vi "CIPT_softwarecontrol auto probe movement 9 8 23 - Copy.vi"() -> ()   [LabVIEW 2022 SP3]
uses:
  Git/CIPT/CIPT/Labview Project/CIPT modes.ctl
  <vilib>/Analysis/baseanly.llb/Mean (DBL).vi
  <vilib>/Utility/file.llb/Read Delimited Spreadsheet (DBL).vi
  <vilib>/Utility/file.llb/Read Delimited Spreadsheet (I64).vi
  <vilib>/gmath/NumericalOptimization/Nonlinear Curve Fit LM.vi
  <vilib>/Utility/file.llb/Write Delimited Spreadsheet (string).vi
  <vilib>/Utility/file.llb/Write Delimited Spreadsheet (I64).vi
  <vilib>/Utility/file.llb/Write Delimited Spreadsheet (DBL).vi
  C:/CIPT/Labview Project/Camera Driver/Labview Driver/OtherDrivers/LabVIEW/ueye.NET/uEyeDotNet.dll
  CIPT/Labview Project/Camera Driver/Labview Driver/OtherDrivers/LabVIEW/ueye.NET/uEyeDotNet.dll
  <vilib>/gmath/NI_Gmath.lvlib
  <instrlib>/Keithley DMM6500 DAQ6500 Series/Keithley DMM6500 DAQ6500 Series.lvlib
  <instrlib>/Keithley 24XX/Keithley 24XX.lvlib
  <instrlib>/Keithley 2182/Keithley 2182.lvlib
  <vilib>/Analysis/NI_AALBase.lvlib
panel:
  out "Resistance":sgl[](array[numeric])
  out "Comms Errors":errorcluster[](array[cluster])
  in  "Save File":bool
  out "error file out":errorcluster
  in  "output file path":path=path "C:/CIPT/Labview Project/csv files/test output.csv"
  in  "stop":bool
  in  "Tab Control":T1(tab)
  in  "Camera ID 3":enum16{"2", "1"}(ring)
  in  "Camera ID 1":enum16{"2", "1"}(ring)
  in  "down a2":bool
  in  "up a2":bool
  in  "down a1":bool
  in  "up a1":bool
  in  "down a3":bool
  in  "up a3":bool
  in  "down all":bool
  in  "up all":bool
  in  "steps /\n continuous \ntoggle":bool
  out "Image first camera":picture
  out "Serial Number 1":string
  in  "Init Camera":bool
  in  "Exit Camera":bool
  in  "Init Camera 2":bool
  in  "Exit Camera 2":bool
  out "Serial Number 2":string
  out "Image second camera":picture
  out "Error Camera 1":errorcluster caption="error"
  out "Error Camera 2":errorcluster caption="error"
  in  "COM 1":refnum<visa-resource-name>="COM1"
  out "error":errorcluster
  in  "Turn On Landing Test":bool
  in  "Step size":i32=10
  in  "Probe Landing File":path=path "C:/CIPT/Labview Project/csv files/Probe Landing cipt.csv"
  out "Probe List":i64[][](array[numeric])
  out "Resistance For Each Relay Setup":sgl[](array[numeric])
  in  "Probe Threshold (ohm)":dbl=100000.0
  out "Touching Probes":i64[][](array[numeric])
  in  "Auto Move Probe To Surface":bool
  out "Loaded":bool
  out "Loaded":bool
  out "Error Probe Configuration File":errorcluster
  in  "Probe Configuration File":path=path "C:/CIPT/Labview Project/csv files/test probe config.csv"
  in  "Probe Settings File":path=path "C:/CIPT/Labview Project/csv files/deafult_probe_setrings.CSV"
  out "Error Probe Settings File":errorcluster
  out "Probe Spacings":dbl[][](array[numeric])
  in  "Load":bool
  in  "Multiplexer":refnum<visa-resource-name>
  out "all rows":i64[][](array[numeric])
  out "Results Description":string[](array[string])
  out "Results":dbl[][](array[numeric])
  out "Probe Set 2":i32
  in  "Compliance voltage (V)":dbl=42.0
  in  "Measure Instrument":refnum<visa-resource-name>
  in  "Radio Buttons":T2 caption="Select Instrumentation"
  in  "Source Instrument":refnum<visa-resource-name>="Sourcemeter"
  in  "Run":bool
  in  "Current (µA)":dbl=10.0
  out "Measurement Log":string
  out "Probe Set":i32
  in  "Measurement Repeats":i32=10
  in  "Size Of Buffer Used For One Measurement":i32=3
  in  "Top Film R est.":dbl=0.25
  in  "Bottm Film R est.":dbl=0.25
  in  "RA est.":dbl=0.25
  out "Top Film R":dbl
  out "Bottom Film R":dbl
  out "RA":dbl
  out "error out (fitting model)":errorcluster
  in  "Fit Data":bool
  out "Measurements Map Out":map{string, dbl[]}(c390)
  # "Probe Landing cipt_probe check: checks probes individually \nProbe Landing cipt: checks for any connection"
  # "All"
  # "End"
  # "home"
  # "Delete"
  # "Insert"
  # "Page Down"
  # "Page up"
  # "F2"
  # "F1"
  # "Steps"
  # "Continuous"
  # "Probe Settings"
  # "Probe Configuration"
  # "I+"
  # "V+"
  # "V-"
  # "I-"
  # "Max Resolution of 2400 is 300 µV in 200 mV range"
  # "/"
  # "Sheet Resistance (RA)"
  # "Estimated Values"
  # "Fitted Values"
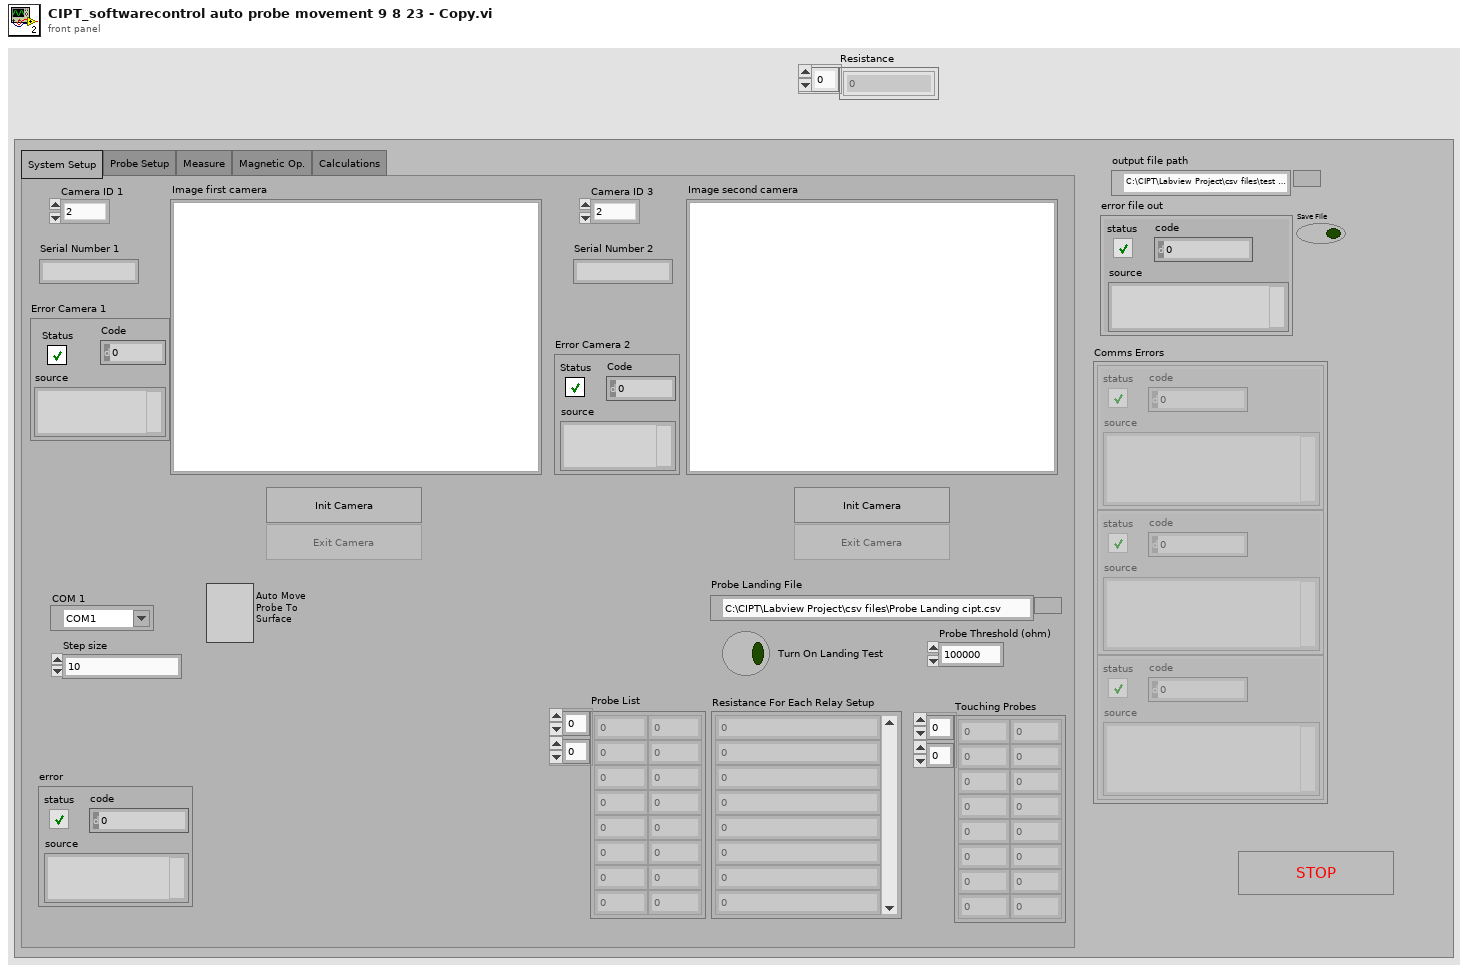
[diagram p1: front panel]
types:
  T1 = enum32{"System Setup", "Probe Setup", "Measure", "Magnetic Op.", "Calculations"}
  T2 = typedef "CIPT modes.ctl" = enum32{"DAQ6510", "2400 Only", "2400 and  2182", "SR830", "SR830 and 6221"}
  T3 = enum32{"System Setup", "Probe Setup", "Measure", "Magnetic Operations", "Calculations + Analyis"}
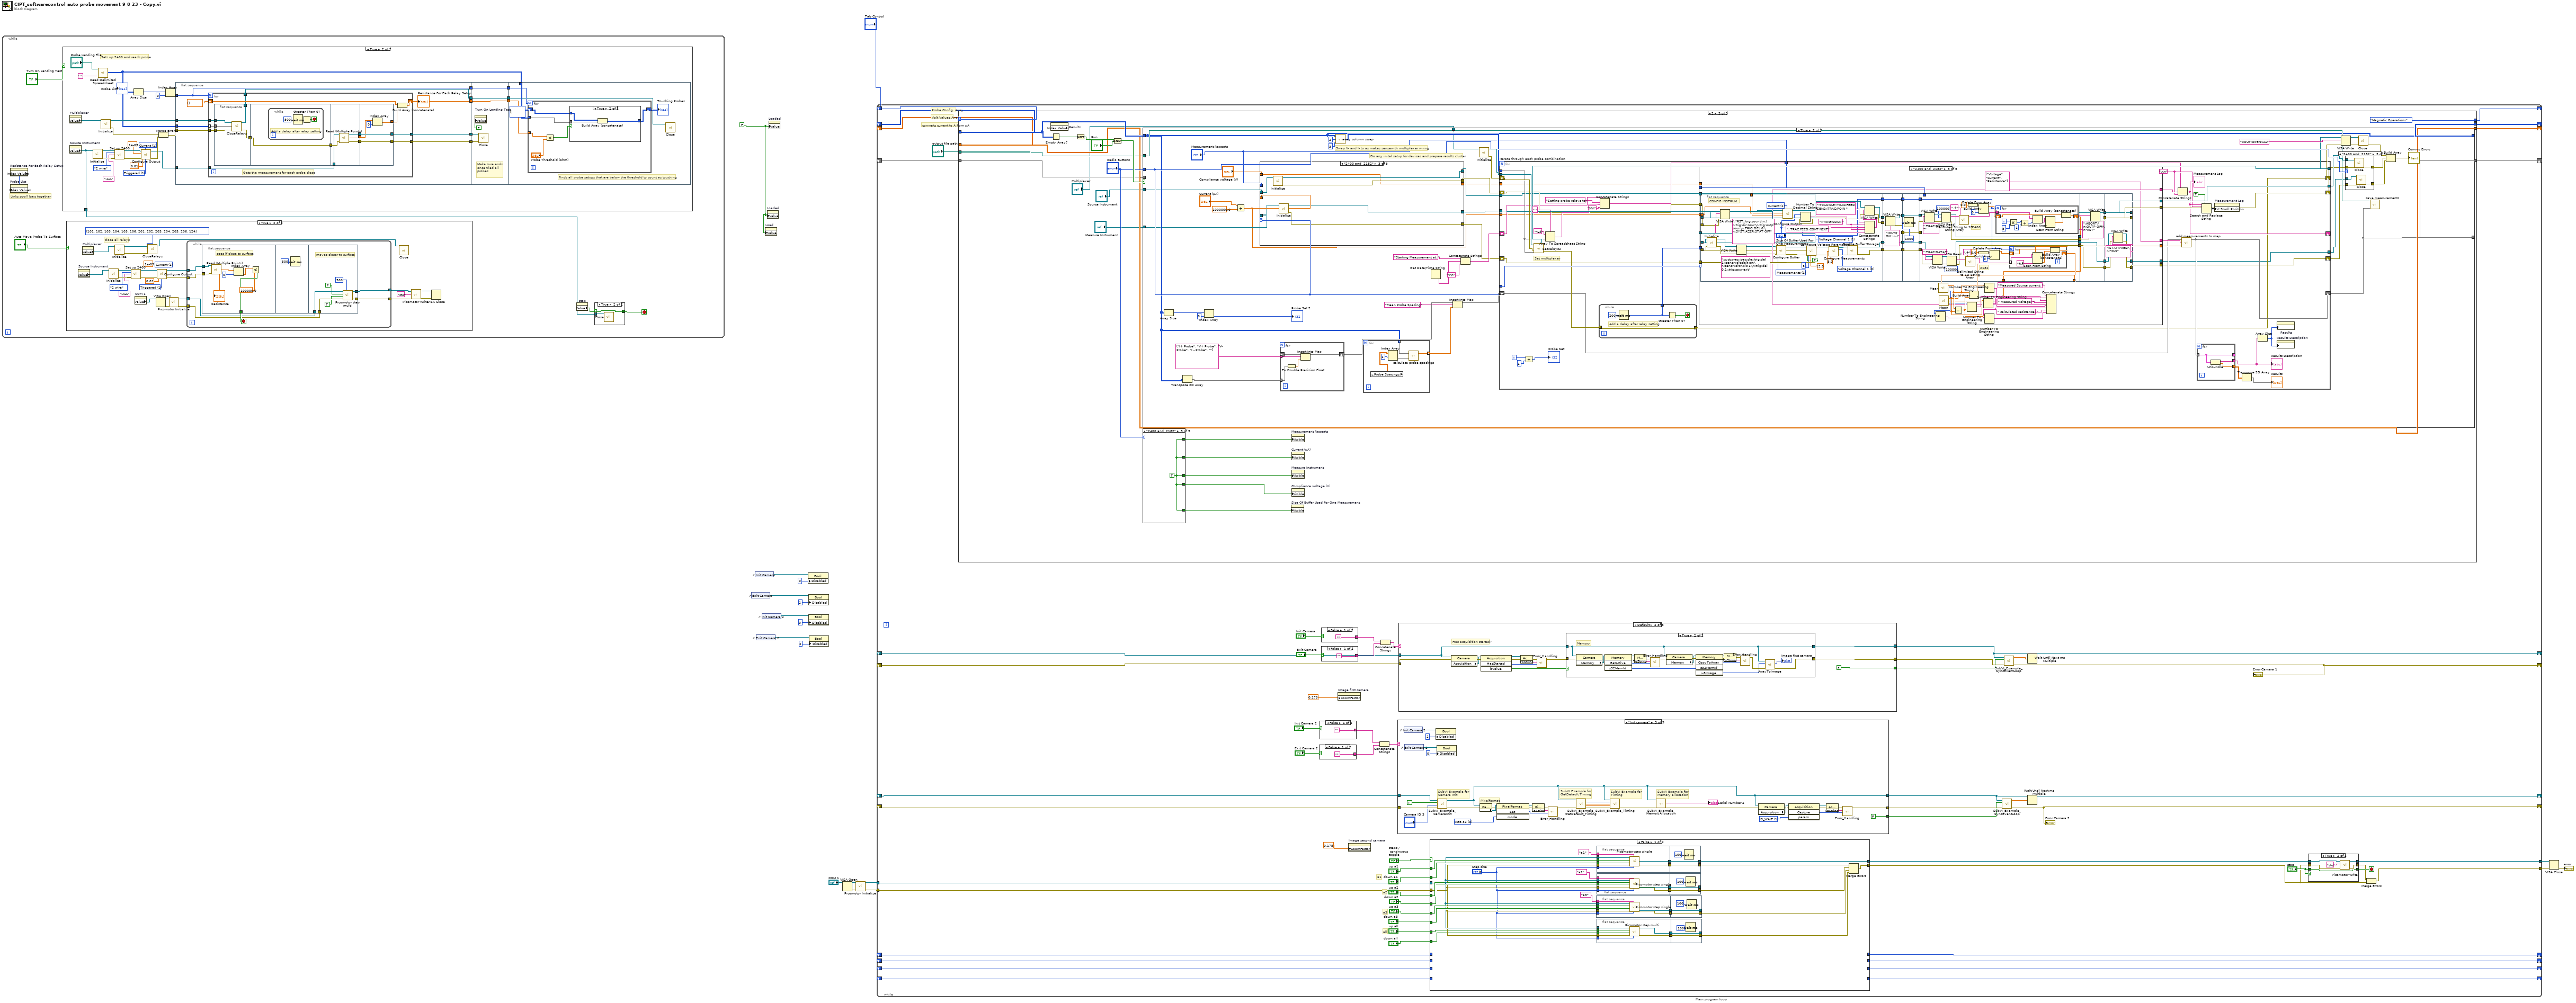
[diagram p0: block diagram]
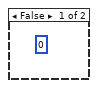
[diagram p4: hidden frame]
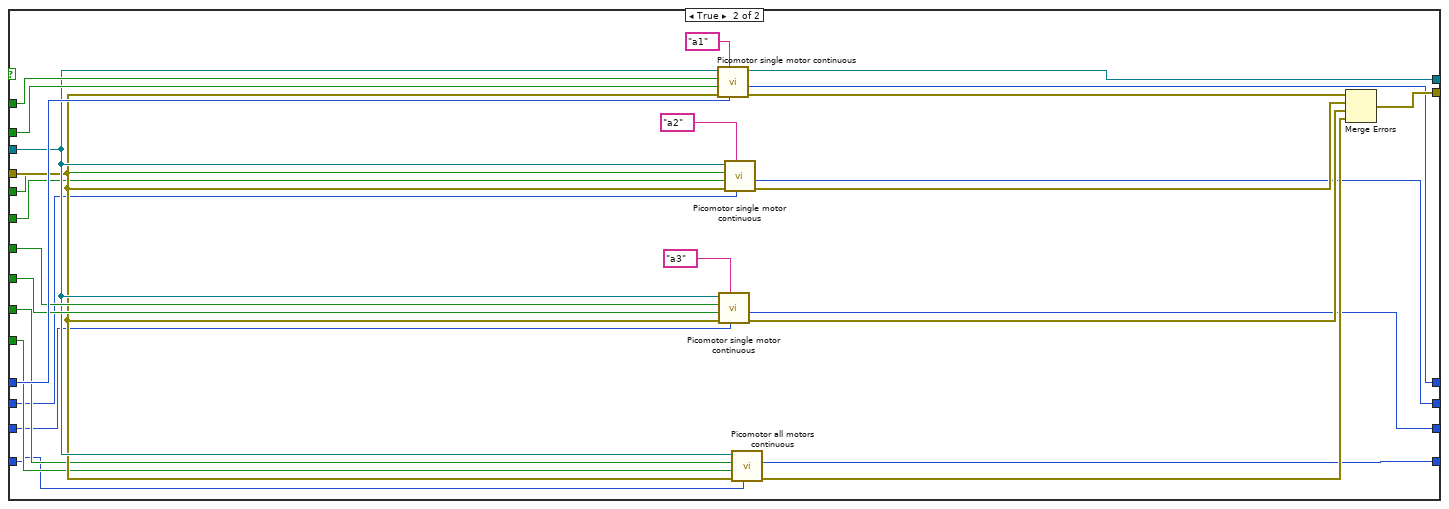
[diagram p6: hidden frame]
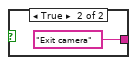
[diagram p8: hidden frame]
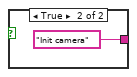
[diagram p9: hidden frame]
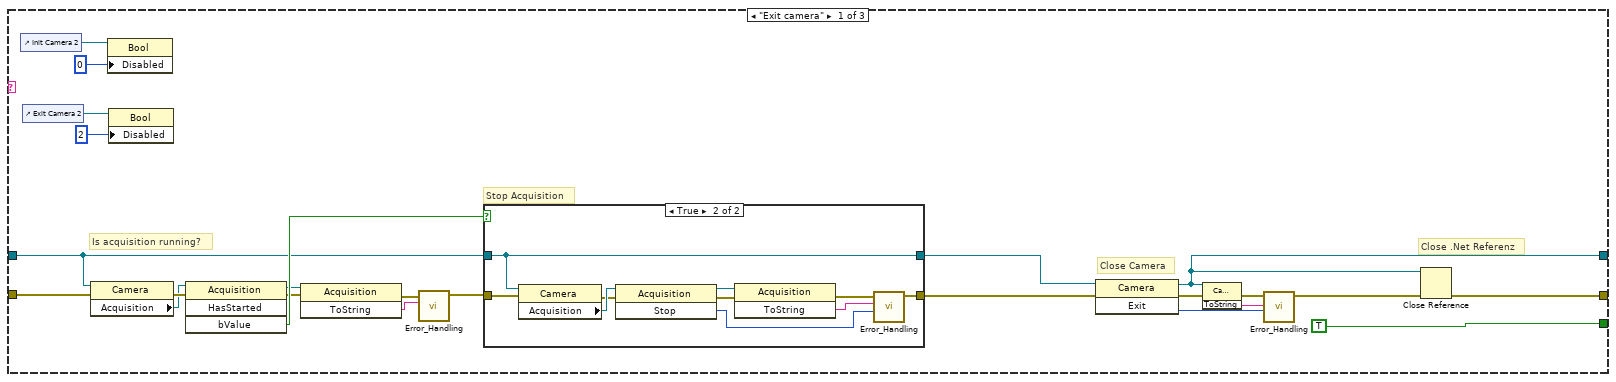
[diagram p10: hidden frame]
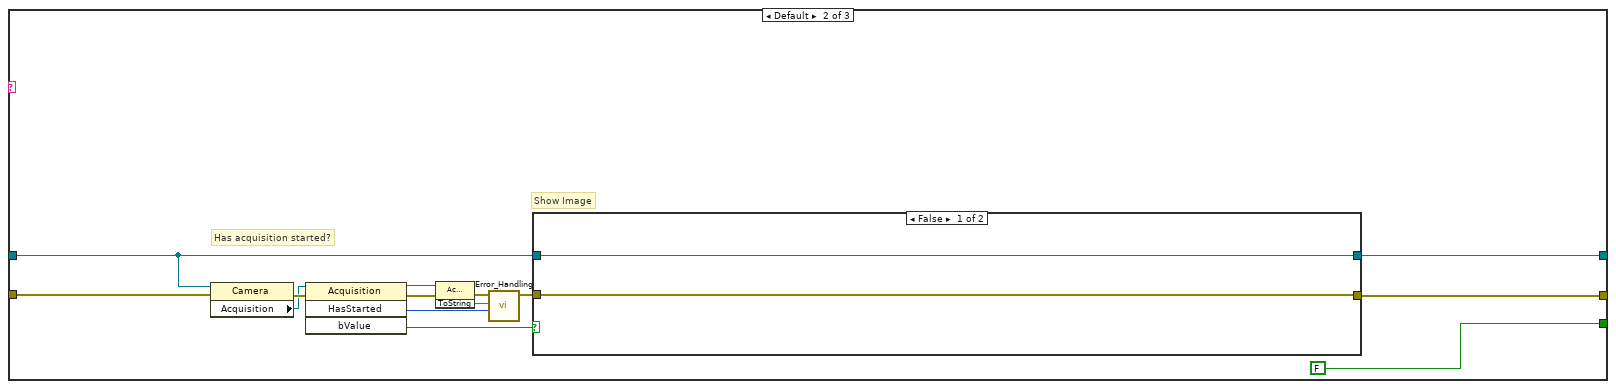
[diagram p12: hidden frame]
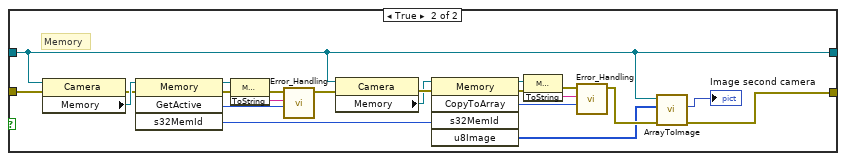
[diagram p13: hidden frame]
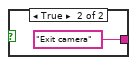
[diagram p14: hidden frame]
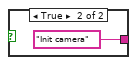
[diagram p15: hidden frame]
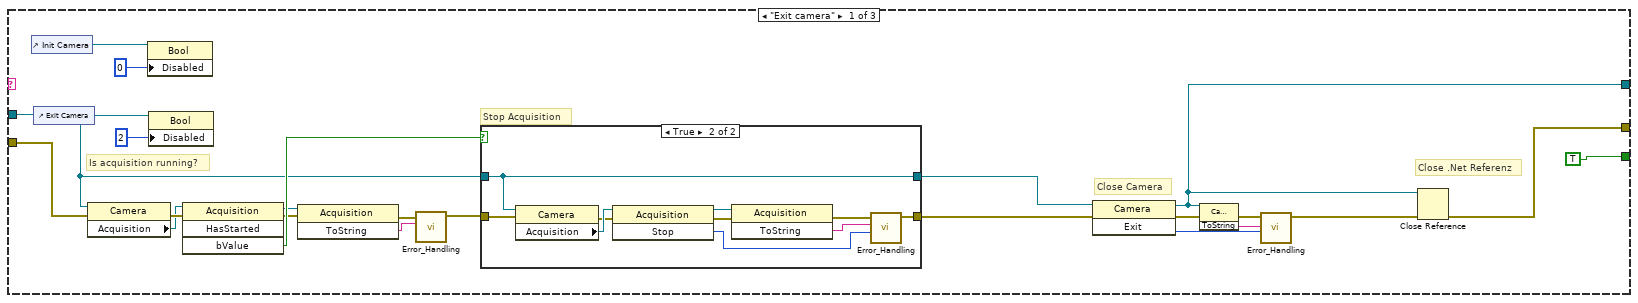
[diagram p16: hidden frame]
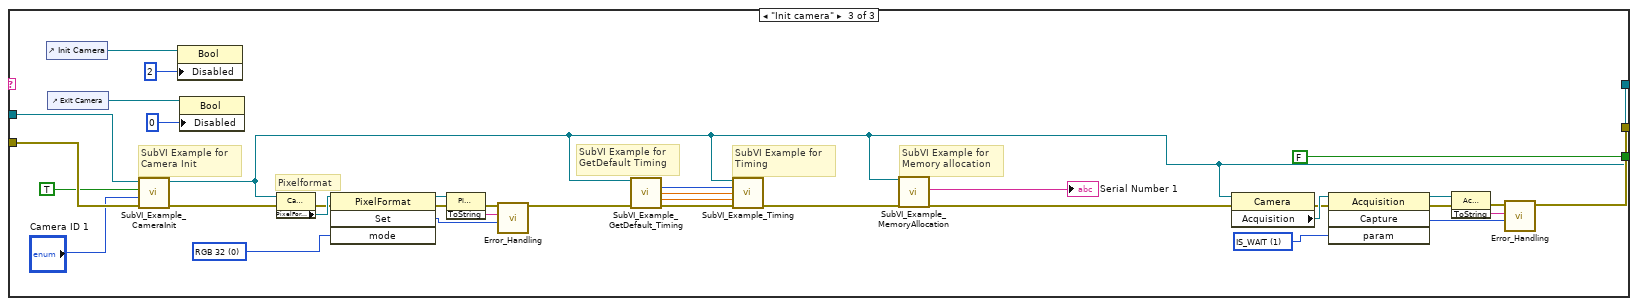
[diagram p19: hidden frame]
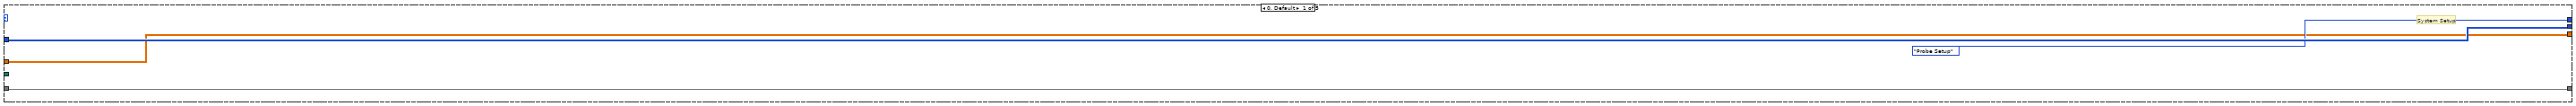
[diagram p20: hidden frame]
diagram:
  w9 = FALSE
  n1 = while {
    stop <- w24 stop-if-true
    # "Links scroll bars together"
    n2 = property on="Resistance For Each Relay Setup" class="Arr (strict)"() -> ("Index Values"=w20:u32[])  [unwired: 2 in, 2 out]
    n3 = property on="Probe List" class="Arr (strict)"("Index Values"=w20) -> ()  [unwired: 2 in, 2 out]
    n4 = case shown="True" "Turn On Landing Test" {
      tunnel: [_ w83] -> w21
      frame False {
        (unwired) 0
      }
      frame True {
        w100 = u16 1 items=["Immediate", "Triggered"] ("Output Type  (0: Immediate)")
        w99 = u16 1 items=["Voltage", "Current"] ("Source Mode  (0: Voltage)")
        # "Sets up 2400 and reads probe"
        n5 = property on="Multiplexer" class="VISAName"() -> ("Value"=w94:refnum<visa-resource-name>)  [unwired: 2 in, 2 out]
        n6 = property on="Source Instrument" class="VISAName"() -> ("Value"=w83:refnum<visa-resource-name>)  [unwired: 2 in, 2 out]
        n7 = call <instrlib>:"Initialize.vi"("VISA resource name"=w83) -> ("error out"=w102:errorcluster, "VISA resource name out"=w101:refnum<visa-resource-name>)  [unwired: 9 in]
        n8 = call-poly <vilib>:"Read Delimited Spreadsheet.vi"("file path (dialog if empty)"="Probe Landing File", "delimiter (\\t)"="," ("delimiter (\\t)")) -> ("all rows"=w80:i64[][])  [unwired: 8 in, 5 out]
        "Probe List" <- w80
        n9 = call <instrlib>:"Initialize.vi"("VISA resource name"=w94) -> ("error out"=w92:errorcluster, "VISA resource name out"=w87:refnum<visa-resource-name>)  [unwired: 9 in]
        n10 = call "Set up 2400.vi"("VISA resource name"=w101, "Sense mode"=enum16{"2 wire", "4 wire"}."2 wire", "Measurement Function"=":ALL", "error in (no error)"=w102) -> ("VISA resource name out"=w103:refnum<visa-resource-name>, "error out"=w104:errorcluster)  [unwired: 10 in]
        n11 = Array Size(array=w80) -> (size(s)=w91:i32[])
        n12 = call <instrlib>:"Configure Output.vi"("Output Type  (0: Immediate)"=w100, "Source Mode  (0: Voltage)"=w99, "error in (no error)"=w104, "Compliance  Level (0.1)"=0.01, "Output Level (0)"=1e-05, "VISA resource name"=w103) -> ("error out"=w93:errorcluster, "VISA resource name out"=w86:refnum<visa-resource-name>)  [unwired: 4 in]
        n13 = Merge Errors(w92, w93) -> (w88:errorcluster)
        n14 = Index Array(array=w91, index=0) -> (element=w89:i32)
        n15 = flat-sequence {
          tunnel: w89 -> [w109]
          tunnel: w88 -> [w116]
          tunnel: w87 -> [w115]
          tunnel: w80 -> [w114]
          tunnel: w86 -> [w113]
          tunnel: [w112] -> w85
          tunnel: [w111] -> w84
          tunnel: [w110] -> w81
          tunnel: [w109] -> w78
          tunnel: [w107] -> w76
          tunnel: w85 -> [w155]
          tunnel: w84 -> [w154]
          tunnel: [w153] -> w82
          tunnel: w81 -> [w153]
          tunnel: [w152] -> w79
          tunnel: w78 -> [w152]
          tunnel: [w151] -> w77
          tunnel: w76 -> [w151]
          tunnel: w82 -> [w162]
          tunnel: w80 -> [w161]
          tunnel: w79 -> [w160]
          tunnel: w77 -> [w157]
          frame #0 {
            n16 = for {
              N: w109 -> [_]
              tunnel: w116 -> [w129]
              tunnel: w115 -> [w128]
              tunnel: w114 -> [w127] mode=indexing
              shift-right: [w122] -> w110
              shift-left: dbl[] [] -> [w121]
              tunnel: w113 -> [w120]
              tunnel: [w119] -> w112
              tunnel: [w118] -> w111
              tunnel: [w117] -> w107
              # "Gets the measurement for each probe close"
              n17 = flat-sequence {
                tunnel: [w136] -> w131
                tunnel: w129 -> [w135]
                tunnel: w128 -> [w134]
                tunnel: w127 -> [w133]
                tunnel: [w132] -> w117
                tunnel: [w137] -> w130
                tunnel: w131 -> [w137]
                tunnel: w130 -> [w145]
                tunnel: [w144] -> w126
                tunnel: [w143] -> w125
                tunnel: [w142] -> w124
                tunnel: w120 -> [w141]
                tunnel: [w149] -> w118
                tunnel: [w150] -> w119
                tunnel: w126 -> [w150]
                tunnel: w125 -> [w149]
                tunnel: w124 -> [w147]
                tunnel: [w146] -> w123
                frame #0 {
                  n18 = call "CloseRelays.vi"("error in (no error)"=w135, "Array"=w133, "VISA Refnum in"=w134) -> ("error out"=w136:errorcluster, "VISA Refnum out"=w132:refnum<visa-resource-name>)  [unwired: 6 in, 1 out]
                }
                frame #1 {
                  n19 = while {
                    stop <- w139 stop-if-true
                    # "Add a delay after relay setting"
                    n20 = Wait (ms)(milliseconds to wait=u32 500) -> (millisecond timer value=w138:u32)
                    n21 = Greater Than 0?(x=w138) -> (x > 0?=w139:bool)
                  }
                }
                frame #2 {
                  n22 = call <instrlib>:"Read (Multiple Points).vi"("VISA resource name"=w141, "error in (no error)"=w145) -> ("VISA resource name out"=w144:refnum<visa-resource-name>, "Resistance"=w142:sgl[], "error out"=w143:errorcluster)  [unwired: 7 in, 4 out]
                }
                frame #3 {
                  n23 = Index Array(array=w147, index=0) -> (element=w146:sgl)
                }
              }
              n24 = Build Array (concatenate)(w121, w123) -> (w122:dbl[])
            }
            "Resistance For Each Relay Setup" <- w110
          }
          frame #1 {
            # "Make sure ends once tried all probes"
            n25 = property on="Turn On Landing Test" class="Bool (strict)"("Value"=FALSE) -> ()  [unwired: 2 in, 2 out]
            n26 = call <instrlib>:"Close.vi"("error in (no error)"=w154, "VISA resource name"=w155) -> ()  [unwired: 9 in, 1 out]
          }
          frame #2 {
            # "Finds all probe setups that are below the threshold to count as touching"
            n27 = for {
              N: w160 -> [_]
              tunnel: w162 -> [w167] mode=indexing
              tunnel: w161 -> [w165] mode=indexing
              shift-right: [w164] -> w159
              shift-left: i64[][] [] -> [w163]
              n28 = Less?(x=w167, y="Probe Threshold (ohm)") -> (x < y?=w166:bool)
              n29 = case shown="True" w166 {
                tunnel: w165 -> [_ w172]
                tunnel: [w169 w171] -> w164
                tunnel: w163 -> [w169 w170]
                frame False {
                }
                frame True {
                  n30 = Build Array (concatenate)(w170, w172) -> (w171:i64[][])
                }
              }
            }
            "Touching Probes" <- w159
            n31 = call <instrlib>:"Close.vi"("VISA resource name"=w157) -> ()  [unwired: 10 in, 1 out]
          }
        }
      }
    }
    n32 = case shown="True" "Auto Move Probe To Surface" {
      frame False {
      }
      frame True {
        (unwired) 1e-05 ("Output Level (0)")
        w46 = u16 1 items=["Immediate", "Triggered"] ("Output Type  (0: Immediate)")
        (unwired) u16 1 items=["Voltage", "Current"] ("Source Mode  (0: Voltage)")
        # "close all relays"
        n33 = property on="Source Instrument" class="VISAName"() -> ("Value"=w42:refnum<visa-resource-name>)  [unwired: 2 in, 2 out]
        n34 = property on="Multiplexer" class="VISAName"() -> ("Value"=w41:refnum<visa-resource-name>)  [unwired: 2 in, 2 out]
        n35 = call <instrlib>:"Initialize.vi"("VISA resource name"=w42) -> ("error out"=w48:errorcluster, "VISA resource name out"=w47:refnum<visa-resource-name>)  [unwired: 9 in]
        n36 = call <instrlib>:"Initialize.vi"("VISA resource name"=w41) -> ("error out"=w38:errorcluster, "VISA resource name out"=w39:refnum<visa-resource-name>)  [unwired: 9 in]
        n37 = call "Set up 2400.vi"("VISA resource name"=w47, "Sense mode"=enum16{"2 wire", "4 wire"}."2 wire", "Measurement Function"=":ALL", "error in (no error)"=w48) -> ("VISA resource name out"=w49:refnum<visa-resource-name>, "error out"=w50:errorcluster)  [unwired: 10 in]
        n38 = property on="COM 1" class="VISAName"() -> ("Value"=w35:refnum<visa-resource-name>)  [unwired: 2 in, 2 out]
        n39 = call "CloseRelays.vi"("error in (no error)"=w38, "Array"=i32[] [101, 102, 103, 104, 105, 106, 201, 202, 203, 204, 205, 206, 124], "VISA Refnum in"=w39) -> ("VISA Refnum out"=w25:refnum<visa-resource-name>)  [unwired: 6 in, 2 out]
        n40 = VISA Open(VISA resource name=w35) -> (VISA resource name=w33:refnum<visa-resource-name>, error out=w34:errorcluster)  [unwired: 4 in]
        n41 = call <instrlib>:"Configure Output.vi"("Output Type  (0: Immediate)"=w46, "error in (no error)"=w50, "Compliance  Level (0.1)"=0.01, "VISA resource name"=w49) -> ("error out"=w36:errorcluster, "VISA resource name out"=w37:refnum<visa-resource-name>)  [unwired: 6 in]
        n42 = call "Picomotor Initialize.vi"("error in (no error)"=w34, "VISA Refnum in"=w33) -> ("error out"=w31:errorcluster, "VISA Refnum out"=w32:refnum<visa-resource-name>)  [unwired: 8 in]
        n43 = while {
          tunnel: w37 -> [w57]
          tunnel: w36 -> [w56]
          tunnel: w32 -> [w54]
          tunnel: w31 -> [w53]
          tunnel: [w52] -> w29
          tunnel: [w51] -> w28
          stop <- w55 stop-if-true
          n44 = flat-sequence {
            tunnel: w57 -> [w62]
            tunnel: w56 -> [w61]
            tunnel: [w60] -> w55
            tunnel: w54 -> [w72]
            tunnel: w53 -> [w71]
            tunnel: [w67] -> w52
            tunnel: [w66] -> w51
            frame #0 {
              # "sees if close to surface"
              n45 = call <instrlib>:"Read (Multiple Points).vi"("VISA resource name"=w62, "error in (no error)"=w61) -> ("Resistance"=w63:sgl[])  [unwired: 7 in, 6 out]
              "Resistance" <- w63
              n46 = Index Array(array=w63, index=0) -> (element=w59:sgl)
              n47 = Less?(x=w59, y=sgl 100000.0 ("x")) -> (x < y?=w60:bool)
            }
            frame #1 {
              n48 = Wait (ms)(milliseconds to wait=u32 500) -> ()  [unwired: 1 out]
            }
            frame #2 {
              # "moves closer to surface"
              n49 = call "Picomotor step multi.vi"("Step size"=500, "error in (no error)"=w71, "down a1"=TRUE, "up a1"=FALSE, "VISA Refnum in"=w72) -> ("error out"=w66:errorcluster, "VISA Refnum out"=w67:refnum<visa-resource-name>)  [unwired: 5 in]
            }
          }
        }
        n50 = call <instrlib>:"Close.vi"("VISA resource name"=w25) -> ()  [unwired: 10 in, 1 out]
        n51 = call "Picomotor Write.vi"("error in (no error)"=w28, "String 3"="sto", "VISA Refnum in"=w29) -> ("error out"=w26:errorcluster, "VISA Refnum out"=w27:refnum<visa-resource-name>)  [unwired: 6 in, 1 out]
        n52 = VISA Close(VISA resource name=w27, error in (no error)=w26) -> ()  [unwired: 1 out]
      }
    }
    n53 = property on="stop" class="Bool (strict)"() -> ("Value"=w22:bool)  [unwired: 2 in, 2 out]
    n54 = case shown="True" w22 {
      selector: w22 -> [w73 w75]
      tunnel: [w73 w75] -> w24
      tunnel: w21 -> [_ w74]
      frame False {
      }
      frame True {
        n55 = call <instrlib>:"Close.vi"("VISA resource name"=w74) -> ()  [unwired: 10 in, 1 out]
      }
    }
  }
  n56 = control-ref of="Exit Camera"() -> (w12:refnum<vi>)
  n57 = control-ref of="Init Camera"() -> (w13:refnum<vi>)
  n58 = control-ref of="Exit Camera 2"() -> (w17:refnum<vi>)
  n59 = control-ref of="Init Camera 2"() -> (w16:refnum<vi>)
  n60 = property on="Load" class="Bool (strict)"("Value"=w9) -> ()  [unwired: 2 in, 2 out]
  n61 = property on="Loaded" class="Bool (strict)"("Value"=w9) -> ()  [unwired: 2 in, 2 out]
  n62 = property on="Loaded" class="Bool (strict)"("Value"=w9) -> ()  [unwired: 2 in, 2 out]
  n63 = property class="Bool"(reference=w13, "Disabled"=u8 0 ("Deaktiviert")) -> ()  [unwired: 1 in, 2 out]
  n64 = property class="Bool"(reference=w12, "Disabled"=u8 2 ("Deaktiviert")) -> ()  [unwired: 1 in, 2 out]
  n65 = property class="Bool"(reference=w16, "Disabled"=u8 0 ("Deaktiviert")) -> ()  [unwired: 1 in, 2 out]
  n66 = property class="Bool"(reference=w17, "Disabled"=u8 2 ("Deaktiviert")) -> ()  [unwired: 1 in, 2 out]
  n67 = VISA Open(VISA resource name="COM 1") -> (VISA resource name=w7:refnum<visa-resource-name>, error out=w6:errorcluster)  [unwired: 4 in]
  n68 = call "Picomotor Initialize.vi"("error in (no error)"=w6, "VISA Refnum in"=w7) -> ("error out"=w4:errorcluster, "VISA Refnum out"=w5:refnum<visa-resource-name>)  [unwired: 8 in]
  n69 = while "Main program loop" {
    shift-right: [w231] -> _
    shift-left: _ -> [w232]
    shift-right: [w230] -> _
    shift-left: "Tab Control" -> [w233]
    shift-right: [w229] -> _
    shift-left: _ -> [w228]
    shift-right: [w226] -> _
    shift-left: _ -> [w225]
    shift-right: [w214] -> _
    shift-left: _ -> [w212]
    shift-right: [w215] -> _
    shift-left: _ -> [w213]
    shift-right: [w202] -> _
    shift-left: _ -> [w200]
    shift-right: [w201] -> _
    shift-left: _ -> [w199]
    tunnel: w5 -> [w186]
    tunnel: w4 -> [w185]
    tunnel: [w198] -> w2
    shift-right: [w183] -> _
    shift-left: _ -> [w179]
    shift-right: [w182] -> _
    shift-left: _ -> [w178]
    shift-right: [w181] -> _
    shift-left: _ -> [w177]
    shift-right: [w180] -> _
    shift-left: _ -> [w176]
    tunnel: [w173] -> w1
    stop <- w197 stop-if-true
    # "a2"
    # "a3"
    # "all"
    # "a1"
    # "converts current to A from µA"
    # "Volt Values Array"
    # "Probe Config. Array"
    n70 = case shown="2" w233 {
      tunnel: w232 -> [w572 w579 w609 w968 w975]
      tunnel: [w572 w583 w608 w968 w975] -> w231
      tunnel: [T3."Probe Setup" ("Tab Control") T3."Measure" ("Tab Control") T3."Magnetic Operations" ("Tab Control") T3."Calculations + Analyis" ("Tab Control") T3."System Setup" ("Tab Control")] -> w230
      tunnel: [w570 w578 w603 w967 w974] -> w229
      tunnel: w228 -> [w570 w577 w603 w967 w974]
      tunnel: "output file path" -> [_ _ w600 _ w973]
      tunnel: [w569 w574 w599 w966 w972] -> w226
      tunnel: w225 -> [w569 w574 w598 w966 w972]
      frame 0, Default {
        # "System Setup"
      }
      frame 1 {
        # "Probe Setup"
        n71 = Empty Array?(array=w579) -> (empty?=w573:bool)
        n72 = Empty Array?(array=w577) -> (empty?=w576:bool)
        n73 = Not(x=w573) -> (.not. x?=→"Loaded":bool)
        n74 = Not(x=w576) -> (.not. x?=→"Loaded":bool)
        n75 = case shown="True" "Load" {
          tunnel: [w585 w586] -> w583
          tunnel: w579 -> [w585 _]
          tunnel: [w584 w587] -> w578
          tunnel: w577 -> [w584 _]
          frame False {
          }
          frame True {
            # "Probe config. file and data aquisition"
            # "Probe settings file and data aquisition"
            n76 = call-poly <vilib>:"Read Delimited Spreadsheet.vi"("file path (dialog if empty)"="Probe Configuration File", "delimiter (\\t)"="," ("delimiter (\\t)")) -> ("all rows"=w586:i64[][], "error out"=→"Error Probe Configuration File":errorcluster)  [unwired: 8 in, 4 out]
            "all rows" <- w586
            n77 = call-poly <vilib>:"Read Delimited Spreadsheet.vi"("file path (dialog if empty)"="Probe Settings File", "delimiter (\\t)"="," ("delimiter (\\t)")) -> ("all rows"=w587:dbl[][], "error out"=→"Error Probe Settings File":errorcluster)  [unwired: 8 in, 4 out]
            "Probe Spacings" <- w587
          }
        }
        n78 = property on="Load" class="Bool (strict)"("Value"=w573) -> ()  [unwired: 2 in, 2 out]
      }
      frame 2 {
        n79 = property on="Results" class="Arr (strict)" props=["Index Values"]() -> ()  [unwired: 2 in, 3 out]
        n80 = Empty Array?(array=w609) -> (empty?=w611:bool)
        n81 = Not(x=w611) -> (.not. x?=w610:bool)
        n82 = Compound Arithmetic op=AND(w610, "Run") -> (w613:bool)
        n83 = case shown="True" w613 {
          tunnel: w609 -> [w624 w643]
          tunnel: [w624 w643] -> w608
          tunnel: "Radio Buttons" -> [_ w669]
          tunnel: w600 -> [_ w657]
          tunnel: [w623 w639] -> w599
          tunnel: w598 -> [w623 _]
          tunnel: "Measure Instrument" -> [_ w631]
          tunnel: "Source Instrument" -> [_ w630]
          tunnel: "Multiplexer" -> [_ w629]
          frame False {
          }
          frame True {
            # "Swap V- and I- to as makes sensewith multiplexer wiring"
            # "Do any inital setup for devices and prepare results cluster"
            n84 = Array Size(array=w643) -> (size(s)=w663:i32[])
            n85 = Transpose 2D Array(2D array=w643) -> (transposed array=w642:i64[][])
            n86 = Index Array "Index Array"(array=w663, index=0) -> (element=→"Probe Set 2":i32)
            n87 = Divide(x="Current (µA)", y=1000000.0) -> (x/y=w625:dbl)
            n88 = case shown="\"2400 and  2182\"" w669 {
              tunnel: w630 -> [_ w707 w713 _ _]
              tunnel: [_ w695 w712 _ _] -> w670
              tunnel: w631 -> [_ _ w714 _ _]
              tunnel: [_ w695 w710 _ _] -> w633
              tunnel: [_ w701 w709 _ _] -> w664
              tunnel: w625 -> [_ w698 _ _ _]
              tunnel: "Compliance voltage (V)" -> [_ w696 w708 _ _]
              tunnel: "Measurement Repeats" -> [_ _ _ _ _]
              tunnel: [_ _ w711 _ _] -> w628
              tunnel: [_ _ w708 _ _] -> w626
              frame "DAQ6510", Default {
              }
              frame "2400 Only" {
                w699 = u16 1 items=["Immediate", "Triggered"] ("Output Type  (0: Immediate)")
                w700 = u16 1 items=["Voltage", "Current"] ("Source Mode  (0: Voltage)")
                n89 = call <instrlib>:"Initialize.vi"("VISA resource name"=w707) -> ("error out"=w705:errorcluster, "VISA resource name out"=w706:refnum<visa-resource-name>)  [unwired: 9 in]
                n90 = call "Set up 2400.vi"("VISA resource name"=w706, "Sense mode"=enum16{"2 wire", "4 wire"}."4 wire", "Measurement Function"=":ALL", "error in (no error)"=w705) -> ("VISA resource name out"=w703:refnum<visa-resource-name>, "error out"=w702:errorcluster)  [unwired: 10 in]
                n91 = call <instrlib>:"Configure Output.vi"("Output Type  (0: Immediate)"=w699, "Source Mode  (0: Voltage)"=w700, "error in (no error)"=w702, "Compliance  Level (0.1)"=w696, "Output Level (0)"=w698, "VISA resource name"=w703) -> ("error out"=w701:errorcluster, "VISA resource name out"=w695:refnum<visa-resource-name>)  [unwired: 4 in]
              }
              frame "2400 and  2182" {
                n92 = call <instrlib>:"Initialize.vi"("VISA resource name"=w713) -> ("error out"=w709:errorcluster, "VISA resource name out"=w710:refnum<visa-resource-name>)  [unwired: 9 in]
                n93 = call <instrlib>:"Initialize.vi"("VISA resource name"=w714) -> ("error out"=w711:errorcluster, "VISA resource name out"=w712:refnum<visa-resource-name>)  [unwired: 9 in]
              }
              frame "SR830" {
              }
              frame "SR830 and 6221" {
              }
            }
            n94 = for {
              tunnel: w642 -> [w681] mode=indexing
              tunnel: string[] ["I+ Probe", "V+ Probe", "V- Probe", "I - Probe", ""] -> [w682] mode=indexing
              shift-right: [w679] -> w647
              shift-left: _ -> [w678]
              n95 = To Double Precision Float(number=w681) -> (double precision float=w680:dbl[])
              n96 = Insert Into Map(map in=w678, key=w682, value=w680) -> (map out=w679:map{string, dbl[]})  [unwired: 2 out]
            }
            n97 = call "array column swap.vi"("Collumn 2 index"=3, "Collumn 1 index"=2, "Input array"=w643) -> ("output array"=w660:i32[][])
            n98 = for {
              tunnel: w643 -> [w674] mode=indexing
              tunnel: [w673] -> w646 mode=indexing
              n99 = local read "Probe Spacings"() -> (w677:dbl[][])
              n100 = Index Array(array=w677, index (row)=1) -> (element=w675:dbl[])  [unwired: 1 in]
              n101 = call "calculate probe spacings.vi"("Probe Spacings"=w675, "Probe list"=w674) -> ("Mean Spacing"=w673:dbl)  [unwired: 1 out]
            }
            n102 = Get Date/Time String() -> (time string=w666:string)  [unwired: 3 in, 1 out]
            n103 = Insert Into Map(map in=w647, key="Mean Probe Spacing", value=w646) -> (map out=w644:map{string, dbl[]})  [unwired: 2 out]
            n104 = Concatenate Strings("Starting Measurement at: ", w666, "\r\n") -> (w655:string)
            n105 = call <instrlib>:"Initialize.vi"("VISA resource name"=w629) -> ("error out"=w671:errorcluster, "VISA resource name out"=w672:refnum<visa-resource-name>)  [unwired: 9 in]
            n106 = for "Iterate through each probe combination" {
              tunnel: w672 -> [w756]
              tunnel: [w755] -> w653
              tunnel: w660 -> [w749] mode=indexing
              tunnel: w669 -> [w754]
              tunnel: w670 -> [w752]
              shift-right: [w738] -> _
              shift-left: w655 -> [w739]
              shift-right: [w750] -> w667
              shift-left: w664 -> [w743]
              shift-right: [w729] -> w639
              shift-left: w644 -> [w731]
              shift-right: [w723] -> w640
              shift-left: w628 -> [w724]
              tunnel: w633 -> [w742]
              tunnel: [w751] -> w668
              shift-right: [w726] -> w635
              shift-left: w671 -> [w753]
              tunnel: [w722] -> w641
              tunnel: "Measurement Repeats" -> [w721]
              tunnel: w626 -> [w717]
              tunnel: w625 -> [w716]
              i -> [w720]
              w736 = "\r\n"
              # "Set multiplexer"
              n107 = Add(x=w720, y=1) -> (x+y=→"Probe Set":i32)
              n108 = call "SetRelays2.vi"("all rows"=w749, "error in (no error)"=w753, "VISA Refnum in"=w756) -> ("error out"=w744:errorcluster, "VISA resource name out"=w755:refnum<visa-resource-name>)  [unwired: 1 in]
              n109 = Array To Spreadsheet String(delimiter (Tab)=",", array=w749, 3:"%d" ("format string")) -> (spreadsheet string=w745:string)
              n110 = while {
                tunnel: [w763] -> w726
                tunnel: w744 -> [w763]
                tunnel: [w760] -> w725
                stop <- w761 stop-if-true
                # "Add a delay after relay setting"
                n111 = Wait (ms)(milliseconds to wait=u32 200) -> (millisecond timer value=w760:u32)
                n112 = Greater Than 0?(x=w760) -> (x > 0?=w761:bool)
              }
              n113 = Concatenate Strings(w739, "Setting probe relays to:", w745, "\r\n") -> (w734:string)
              n114 = case shown="\"2400 and  2182\"" w754 {
                tunnel: w752 -> [w765 w769 w834 w958 w962]
                tunnel: w742 -> [w764 w790 w842 w959 w963]
                tunnel: w743 -> [w766 w789 w841 w960 w964]
                tunnel: [w764 w787 w802 w959 w963] -> w751
                tunnel: [w766 w786 w810 w960 w964] -> w750
                tunnel: [_ w779 w835 _ _] -> w740
                tunnel: w721 -> [_ w778 w840 _ _]
                tunnel: [_ w772 w839 _ _] -> w732
                tunnel: [_ string[] ["Voltage", "Current", "Resistance"] string[] ["Voltage", "Current", "Resistance"] _ _] -> w733
                tunnel: w725 -> [_ _ _ _ _]
                tunnel: w724 -> [w767 w770 w833 w961 w965]
                tunnel: [w767 w770 w806 w961 w965] -> w723
                tunnel: [w765 w769 w803 w958 w962] -> w722
                tunnel: w717 -> [_ _ w795 _ _]
                tunnel: w716 -> [_ _ w794 _ _]
                frame "DAQ6510", Default {
                }
                frame "2400 Only" {
                  w788 = u16 0 items=["Fixed", "Sweep", "List"] ("Output Mode (0: Fixed)")
                  n115 = call <instrlib>:"Read (Multiple Points).vi"("VISA resource name"=w790, "Sample Count (1)"=w778, "error in (no error)"=w789, "Output Mode (0: Fixed)"=w788) -> ("Voltage"=w768:sgl[], "VISA resource name out"=w787:refnum<visa-resource-name>, "Current"=w777:sgl[], "Resistance"=w776:sgl[], "error out"=w786:errorcluster)  [unwired: 5 in, 2 out]
                  n116 = call-poly <vilib>:"Mean.vi"("X"=w768) -> ("mean"=w775:dbl)  [unwired: 1 out]
                  n117 = call-poly <vilib>:"Mean.vi"("X"=w777) -> ("mean"=w774:dbl)  [unwired: 1 out]
                  n118 = call-poly <vilib>:"Mean.vi"("X"=w776) -> ("mean"=w773:dbl)  [unwired: 1 out]
                  n119 = Build Array(w775, w774, w773) -> (w772:dbl[])
                  n120 = Number To Engineering String(4:w775) -> (0:w780:string)  [unwired: 3 in]
                  n121 = Number To Engineering String(4:w774) -> (0:w784:string)  [unwired: 3 in]
                  n122 = Number To Engineering String(4:w773) -> (0:w781:string)  [unwired: 3 in]
                  n123 = Concatenate Strings("Measured I = ", w784, " V = " ("string"), w780, "R = " ("string"), w781) -> (w779:string)
                }
                frame "2400 and  2182" {
                  n124 = flat-sequence {
                    tunnel: w833 -> [w849]
                    tunnel: w834 -> [w850]
                    tunnel: w841 -> [w851]
                    tunnel: w842 -> [w852]
                    tunnel: [w856] -> w805
                    tunnel: [w855] -> w804
                    tunnel: [w854] -> w797
                    tunnel: [w853] -> w796
                    tunnel: w795 -> [w847]
                    tunnel: w794 -> [w846]
                    tunnel: ["Size Of Buffer Used For One Measurement"] -> w791
                    tunnel: [w889] -> w822
                    tunnel: [w888] -> w820
                    tunnel: [w886] -> w817
                    tunnel: [w885] -> w815
                    tunnel: w805 -> [w889]
                    tunnel: w804 -> [w888]
                    tunnel: w797 -> [w887]
                    tunnel: w796 -> [_]
                    tunnel: [w883] -> w792
                    tunnel: w791 -> [w883]
                    tunnel: w822 -> [w895]
                    tunnel: [w895] -> w821
                    tunnel: w820 -> [w894]
                    tunnel: [w894] -> w819
                    tunnel: [w892] -> w818
                    tunnel: w817 -> [w892]
                    tunnel: [w891] -> w816
                    tunnel: w815 -> [w891]
                    tunnel: [w890] -> w793
                    tunnel: w792 -> [w890]
                    tunnel: w840 -> [_]
                    tunnel: w821 -> [w905]
                    tunnel: w819 -> [w904]
                    tunnel: w818 -> [w907]
                    tunnel: w816 -> [w906]
                    tunnel: [w903] -> w814
                    tunnel: [w902] -> w813
                    tunnel: [w900] -> w812
                    tunnel: [w899] -> w811
                    tunnel: [w898] -> w808
                    tunnel: [w897] -> w807
                    tunnel: w793 -> [w896]
                    tunnel: w812 -> [w950]
                    tunnel: w811 -> [w949]
                    tunnel: w808 -> [w945]
                    tunnel: w807 -> [w946]
                    tunnel: [w947] -> w801
                    tunnel: [w946] -> w800
                    tunnel: [w945] -> w799
                    tunnel: [w944] -> w798
                    tunnel: [w956] -> w802
                    tunnel: [w951] -> w803
                    tunnel: [w952] -> w806
                    tunnel: [w957] -> w810
                    tunnel: w801 -> [w957]
                    tunnel: w800 -> [w953]
                    tunnel: w799 -> [w954]
                    tunnel: w798 -> [w956]
                    frame #0 {
                      w860 = 0 items=["Voltage Channel 1", "Voltage Channel 2", "Temperature Channel 1", "Temperature Channel 2"] ("Measurement (0: Voltage Channel 1)")
                      w848 = u16 1 items=["Voltage", "Current"] ("Source Mode  (0: Voltage)")
                      w873 = 1 items=["Voltage Channel 1"=1, "Voltage Channel 2"=2] ("Measurement (1: Voltage Channel 1)")
                      w874 = 1 items=["None", "Measurements", "Math Calculation"] ("Buffer Source (0: None)")
                      # "CONFIG INSTRUM"
                      n125 = call <instrlib>:"Initialize.vi"("error in (no error)"=w849, "VISA resource name"=w850) -> ("error out"=w858:errorcluster, "VISA resource name out"=w859:refnum<visa-resource-name>)  [unwired: 8 in]
                      n126 = VISA Write(VISA resource name=w852, write buffer=":*RST;:trig:sour tlin;\n:trig:dir sour;\n:trig:outp sour;\n:TRIG:DEL 0;\n:SYST:AZER:STAT OFF", error in (no error)=w851) -> (VISA resource name out=w869:refnum<visa-resource-name>, error out=w864:errorcluster)  [unwired: 1 out]
                      n127 = VISA Write(VISA resource name=w859, write buffer=":syst:pres;:trac:cle;:trig:del 1;:sens:volt:delt on;\n:sens:volt:nplc 1;\n:trig:del 0.1;:trig:sour ext", error in (no error)=w858) -> (VISA resource name out=w871:refnum<visa-resource-name>, error out=w870:errorcluster)  [unwired: 1 out]
                      n128 = call <instrlib>:"Configure Buffer.vi"("error in (no error)"=w870, "Buffer Source (0: None)"=w874, "Buffer Size (2)"="Size Of Buffer Used For One Measurement", "VISA resource name"=w871) -> ("error out"=w875:errorcluster, "VISA resource name out"=w878:refnum<visa-resource-name>)  [unwired: 6 in]
                      n129 = call <instrlib>:"Configure Output.vi"("Source Mode  (0: Voltage)"=w848, "error in (no error)"=w864, "Compliance  Level (0.1)"=w847, "Output Level (0)"=w846, "VISA resource name"=w869) -> ("error out"=w863:errorcluster, "VISA resource name out"=w845:refnum<visa-resource-name>)  [unwired: 5 in]
                      n130 = Number To Decimal String(number="Size Of Buffer Used For One Measurement") -> (decimal integer string=w865:string)  [unwired: 1 in]
                      n131 = call <instrlib>:"Configure Voltage Parameters.vi"("VISA resource name"=w878, "Measurement (1: Voltage Channel 1)"=w873, "Voltage Resolution (8)"=8, "Range Value (12)"=12.0, "Autorange (T: Enable)"=TRUE, "error in (no error)"=w875) -> ("VISA resource name out"=w877:refnum<visa-resource-name>, "error out"=w876:errorcluster)  [unwired: 8 in]
                      n132 = call <instrlib>:"Configure Measurements.vi"("VISA resource name"=w877, "Measurement (0: Voltage Channel 1)"=w860, "Integration Rate (5)"=5.0, "error in (no error)"=w876) -> ("VISA resource name out"=w862:refnum<visa-resource-name>, "error out"=w861:errorcluster)  [unwired: 10 in]
                      n133 = call <instrlib>:"Enable Buffer Storage.vi"("error in (no error)"=w861, "VISA resource name"=w862) -> ("error out"=w855:errorcluster, "VISA resource name out"=w856:refnum<visa-resource-name>)  [unwired: 8 in]
                      n134 = Concatenate Strings(":TRAC:CLE;:TRAC:FEED SENS;:TRAC:POIN " ("write buffer"), w865, ";:TRIG:COUN " ("write buffer"), w865, ";:TRAC:FEED:CONT NEXT" ("write buffer")) -> (w844:string)
                      n135 = VISA Write(VISA resource name=w845, write buffer=w844, error in (no error)=w863) -> (VISA resource name out=w854:refnum<visa-resource-name>, error out=w853:errorcluster)  [unwired: 1 out]
                    }
                    frame #1 {
                      n136 = VISA Write(VISA resource name=w887, write buffer=":OUTP ON;:init") -> (VISA resource name out=w886:refnum<visa-resource-name>, error out=w885:errorcluster)  [unwired: 1 in, 1 out]
                    }
                    frame #2 {
                      n137 = Wait (ms)(milliseconds to wait=u32 1000) -> ()  [unwired: 1 out]
                    }
                    frame #3 {
                      # "2182"
                      # "2400"
                      n138 = VISA Write(VISA resource name=w907, write buffer=":TRAC:DATA?", error in (no error)=w906) -> (VISA resource name out=w917:refnum<visa-resource-name>, error out=w916:errorcluster)  [unwired: 1 out]
                      n139 = VISA Write(VISA resource name=w905, write buffer=":TRAC:DATA?", error in (no error)=w904) -> (VISA resource name out=w926:refnum<visa-resource-name>, error out=w925:errorcluster)  [unwired: 1 out]
                      n140 = VISA Read(VISA resource name=w917, byte count=u32 100000, error in (no error)=w916) -> (VISA resource name out=w900:refnum<visa-resource-name>, read buffer=w913:string, error out=w899:errorcluster)  [unwired: 1 out]
                      n141 = VISA Read(VISA resource name=w926, byte count=u32 100000, error in (no error)=w925) -> (VISA resource name out=w898:refnum<visa-resource-name>, read buffer=w923:string, error out=w897:errorcluster)  [unwired: 1 out]
                      n142 = call <vilib>:"Delimited String to 1D String Array.vi"("delimiter"=",+" ("delimiter (Tab)"), "delimited string"=w913) -> ("string array"=w909:string[])  [unwired: 9 in]
                      n143 = call <vilib>:"Delimited String to 1D String Array.vi"("delimiter"=",+" ("delimiter (Tab)"), "delimited string"=w923) -> ("string array"=w918:string[])  [unwired: 9 in]
                      n144 = Build Array(0.0 ("array")) -> (w911:dbl[])
                      n145 = Build Array(0.0 ("array")) -> (w921:dbl[])
                      n146 = Delete From Array(array=w911, index=0) -> (array with subset deleted=w901:dbl[])  [unwired: 1 in, 1 out]
                      n147 = Delete From Array(array=w921, index=0) -> (array with subset deleted=w919:dbl[])  [unwired: 1 in, 1 out]
                      n148 = for {
                        N: w896 -> [_]
                        shift-right: [w932] -> w902
                        shift-left: w901 -> [w931]
                        tunnel: w909 -> [w930]
                        i -> [w938]
                        n149 = Multiply(x=w938, y=5) -> (x*y=w937:i32)
                        n150 = Add(x=w937, y=1) -> (x+y=w934:i32)
                        n151 = Index Array(array=w930, index=w934) -> (element=w929:string)
                        n152 = Scan From String(input string=w929) -> (output 1=w933:dbl)  [unwired: 4 in, 3 out]
                        n153 = Build Array (concatenate)(w931, w933) -> (w932:dbl[])
                      }
                      n154 = for {
                        N: w896 -> [_]
                        shift-right: [w941] -> w903
                        shift-left: w919 -> [w940]
                        tunnel: w918 -> [w939] mode=indexing
                        n155 = Scan From String(format string="%f", input string=w939) -> (output 1=w942:dbl)  [unwired: 3 in, 3 out]
                        n156 = Build Array (concatenate)(w940, w942) -> (w941:dbl[])
                      }
                    }
                    frame #4 {
                      n157 = VISA Write(VISA resource name=w950, write buffer=":ABORT;\n:OUTP OFF;\n*RST" ("data"), error in (no error)=w949) -> (VISA resource name out=w944:refnum<visa-resource-name>, error out=w947:errorcluster)  [unwired: 1 out]
                    }
                    frame #5 {
                      n158 = VISA Write(VISA resource name=w954, write buffer=":STAT:PRES;\n:*CLS" ("data"), error in (no error)=w953) -> (VISA resource name out=w951:refnum<visa-resource-name>, error out=w952:errorcluster)  [unwired: 1 out]
                    }
                  }
                  n159 = call-poly <vilib>:"Mean.vi"("X"=w814) -> ("mean"=w838:dbl, "error"=w826:i32)
                  n160 = Number To Engineering String(4:w826) -> (0:w825:string)  [unwired: 3 in]
                  n161 = call-poly <vilib>:"Mean.vi"("X"=w813) -> ("mean"=w837:dbl, "error"=w830:i32)
                  n162 = Divide(x=w838, y=w837) -> (x/y=w836:dbl)
                  n163 = Number To Engineering String(4:w830) -> (0:w829:string)  [unwired: 3 in]
                  n164 = Build Array(w838, w837, w836) -> (w839:dbl[])
                  n165 = Number To Engineering String(4:w837) -> (0:w831:string)  [unwired: 3 in]
                  n166 = Number To Engineering String(4:w836) -> (0:w823:string)  [unwired: 3 in]
                  n167 = Number To Engineering String(4:w838) -> (0:w827:string)  [unwired: 3 in]
                  n168 = Concatenate Strings("Measured Source current: " ("string"), w831, w829, " measured voltage: " ("string"), w827, w825, " calculated resistance: " ("string"), w823) -> (w835:string)
                }
                frame "SR830" {
                }
                frame "SR830 and 6221" {
                }
              }
              n169 = Concatenate Strings(w734, w740, w736) -> (w738:string)
              "Measurement Log" <- w738
              n170 = call "add measurements to map.vi"("Measurement Values"=w732, "Measurement Names"=w733, "Measurements Map in"=w731) -> ("Measurements Map Out"=w729:map{string, dbl[]})  [unwired: 2 in]
              n171 = for {
                tunnel: [w759] -> _ mode=indexing
                tunnel: w729 -> [w759] mode=indexing
                tunnel: [w758] -> w728 mode=indexing
                tunnel: [w757] -> w727 mode=indexing
                n172 = Unbundle(w759) -> (w758:string, "Array"=w757:dbl[])
              }
              "Results Description" <- w728
              n173 = Search and Replace String(replace all?=TRUE, input string=w738, search string=w736) -> (number of replacements=w735:i32)  [unwired: 5 in, 3 out]
              n174 = property on="Measurement Log" class="Str"("Text.Scroll Position"=w735) -> ()  [unwired: 2 in, 2 out]
              n175 = Transpose 2D Array(2D array=w727) -> (transposed array=→"Results":dbl[][])
              n176 = Array Size(array=w728) -> (size(s)=w730:i32)
              n177 = property on="Results" class="Arr (strict)"("Number of Columns"=w730) -> ()  [unwired: 2 in, 2 out]
              n178 = property on="Results Description" class="Arr (strict)"("Number of Columns"=w730) -> ()  [unwired: 2 in, 2 out]
            }
            n179 = VISA Write(VISA resource name=w653, write buffer="ROUT:OPEN:ALL", error in (no error)=w635) -> (VISA resource name out=w652:refnum<visa-resource-name>, error out=w651:errorcluster)  [unwired: 1 out]
            n180 = case shown="\"2400 and  2182\"" w669 {
              tunnel: w668 -> [_ w688 w693 _ _]
              tunnel: w667 -> [w684 w687 w694 _ _]
              tunnel: [w684 w686 w689 _ _] -> w638
              tunnel: w641 -> [_ _ w692 _ _]
              tunnel: w640 -> [w683 w685 w691 _ _]
              tunnel: [w683 w685 w690 _ _] -> w637
              frame "DAQ6510", Default {
              }
              frame "2400 Only" {
                n181 = call <instrlib>:"Close.vi"("error in (no error)"=w687, "VISA resource name"=w688) -> ("error out"=w686:errorcluster)  [unwired: 9 in]
              }
              frame "2400 and  2182" {
                n182 = call <instrlib>:"Close.vi"("error in (no error)"=w694, "VISA resource name"=w693) -> ("error out"=w689:errorcluster)  [unwired: 9 in]
                n183 = call <instrlib>:"Close.vi"("error in (no error)"=w691, "VISA resource name"=w692) -> ("error out"=w690:errorcluster)  [unwired: 9 in]
              }
              frame "SR830" {
              }
              frame "SR830 and 6221" {
              }
            }
            n184 = call <instrlib>:"Close.vi"("error in (no error)"=w651, "VISA resource name"=w652) -> ("error out"=w634:errorcluster)  [unwired: 9 in]
            n185 = call "save measurements.vi"("Save path"=w657, "Measurements In"=w639) -> ()  [unwired: 12 in, 2 out]
            n186 = Build Array(w634, w638, w637) -> (→"Comms Errors":errorcluster[])
          }
        }
        n187 = case shown="\"2400 and  2182\"" "Radio Buttons" {
          tunnel: [w614 w616 w618 w619 w622] -> w607
          tunnel: [w614 w617 w618 w619 w621] -> w606
          tunnel: [TRUE w617 w618 TRUE w622] -> w602
          tunnel: [w614 w617 w618 w619 w622] -> w601
          tunnel: [w614 w616 w618 w619 w621] -> w594
          frame "DAQ6510", Default {
            w614 = FALSE
          }
          frame "2400 Only" {
            w617 = TRUE
            w616 = FALSE
          }
          frame "2400 and  2182" {
            w618 = TRUE
          }
          frame "SR830" {
            w619 = FALSE
          }
          frame "SR830 and 6221" {
            w621 = FALSE
            w622 = TRUE
          }
        }
        n188 = property on="Size Of Buffer Used For One Measurement" class="DigNum (strict)"("Visible"=w594) -> ()  [unwired: 2 in, 2 out]
        n189 = property on="Measurement Repeats" class="DigNum (strict)"("Visible"=w602) -> ()  [unwired: 2 in, 2 out]
        n190 = property on="Current (µA)" class="DigNum (strict)"("Visible"=w606) -> ()  [unwired: 2 in, 2 out]
        n191 = property on="Measure Instrument" class="VISAName"("Visible"=w607) -> ()  [unwired: 2 in, 2 out]
        n192 = property on="Compliance voltage (V)" class="DigNum (strict)"("Visible"=w601) -> ()  [unwired: 2 in, 2 out]
      }
      frame 3 {
        # "Magnetic Op."
      }
      frame 4 {
        # "Calculations"
        # "Save File - saves collected data into a (csv) file and asks for a file path if not already given"
        n193 = Look In Map(map=w972, key="Resistance") -> (value=w970:dbl[])  [unwired: 1 in, 1 out]
        n194 = Build Array("Top Film R est.", "Bottm Film R est.", "RA est.") -> (w980:dbl[])
        n195 = case shown="True" "Fit Data" {
          tunnel: w975 -> [_ w1000]
          tunnel: w980 -> [_ w998]
          tunnel: [dbl[] [0.0, 0.0, 0.0] w989] -> w977
          tunnel: w970 -> [_ w987]
          frame False {
          }
          frame True {
            # "Calculated R"
            # "Mean probe spacing"
            n196 = Index Array(array=w1000, index (col)=4 ("disabled index (col)")) -> (element=w999:i64[])  [unwired: 1 in]
            n197 = vi-ref "modelFunction.vi"() -> (w997:refnum<vi>)
            n198 = call-poly <vilib>:"Nonlinear Curve Fit.vi"("Y"=w987, "f(x,a)"=w997, "X"=w999, "initial parameters"=w998) -> ("best fit parameters"=w989:dbl[], "error out"=→"error out (fitting model)":errorcluster)  [unwired: 6 in, 4 out]
            n199 = Index Array(array=w989, index=0) -> (element=→"Top Film R":dbl)
            n200 = Index Array(array=w989, index=1) -> (element=→"Bottom Film R":dbl)
            n201 = Index Array(array=w989, index=2) -> (element=→"RA":dbl)
          }
        }
        n202 = case shown="True" "Save File" {
          tunnel: w975 -> [_ w1021]
          tunnel: string[] ["I+", "V+", "V-", "I-", "x (mean probe spacing)", "V", "I (µA)", "R (=V/I)"] -> [_ w1017]
          tunnel: string[] ["R (t)", "R (b)", "RA"] -> [_ w1009]
          tunnel: w977 -> [_ w1002]
          tunnel: w973 -> [_ w1001]
          frame False {
          }
          frame True {
            n203 = call-poly <vilib>:"Write Delimited Spreadsheet.vi"("file path (dialog if empty)"=w1001, "1D data"=w1017, "delimiter (\\t)"="," ("delimiter (\\t)")) -> ("new file path (Not A Path if cancelled)"=w1019:path, "error out"=w1018:errorcluster)  [unwired: 11 in]
            n204 = call-poly <vilib>:"Write Delimited Spreadsheet.vi"("file path (dialog if empty)"=w1019, "format (%d)"="%.6f" ("format (%.3f)"), "2D data"=w1021, "append to file? (new file:F)"=TRUE, "error in (no error)"=w1018, "delimiter (\\t)"="," ("delimiter (\\t)")) -> ("new file path (Not A Path if cancelled)"=w1011:path, "error out"=w1010:errorcluster)  [unwired: 8 in]
            n205 = call-poly <vilib>:"Write Delimited Spreadsheet.vi"("file path (dialog if empty)"=w1011, "format (%s)"="%.6f" ("format (%.3f)"), "1D data"=w1009, "append to file? (new file:F)"=TRUE, "error in (no error)"=w1010, "delimiter (\\t)"="," ("delimiter (\\t)")) -> ("new file path (Not A Path if cancelled)"=w1004:path, "error out"=w1003:errorcluster)  [unwired: 8 in]
            n206 = call-poly <vilib>:"Write Delimited Spreadsheet.vi"("file path (dialog if empty)"=w1004, "format (%.3f)"="%.6f", "1D data"=w1002, "append to file? (new file:F)"=TRUE, "error in (no error)"=w1003, "delimiter (\\t)"="," ("delimiter (\\t)")) -> ("error out"=→"error file out":errorcluster)  [unwired: 8 in, 1 out]
          }
        }
        "Measurements Map Out" <- w972
      }
    }
    n207 = case shown="False" "Exit Camera 2" {
      tunnel: ["" "Exit camera"] -> w207
      frame False {
      }
      frame True {
      }
    }
    n208 = case shown="False" "Init Camera 2" {
      tunnel: ["" "Init camera"] -> w210
      frame False {
      }
      frame True {
      }
    }
    n209 = case shown="False" "Init Camera" {
      tunnel: ["" "Init camera"] -> w223
      frame False {
      }
      frame True {
      }
    }
    n210 = case shown="False" "Exit Camera" {
      tunnel: ["" "Exit camera"] -> w220
      frame False {
      }
      frame True {
      }
    }
    n211 = property on="Image first camera" class="Pict"("ZoomFactor"=0.175) -> ()  [unwired: 2 in, 2 out]
    n212 = property on="Image second camera" class="Pict"("ZoomFactor"=0.175) -> ()  [unwired: 2 in, 2 out]
    n213 = Concatenate Strings(w210, w207) -> (w209:string)
    n214 = Concatenate Strings(w223, w220) -> (w222:string)
    n215 = case shown="\"Init camera\"" w209 {
      tunnel: w200 -> [w351 w382 w447]
      tunnel: w199 -> [w352 w381 w446]
      tunnel: [w361 w384 w425] -> w202
      tunnel: [w362 w383 w426] -> w206
      tunnel: [TRUE FALSE FALSE] -> w204
      frame "Exit camera" {
        # "Close .Net Referenz"
        # "Is acquisition running?"
        # "Stop Acquisition"
        # "Close Camera"
        n216 = control-ref of="Init Camera 2"() -> (w346:refnum<vi>)
        n217 = control-ref of="Exit Camera 2"() -> (w345:refnum<vi>)
        n218 = property class="Camera"(reference=w351, error in=w352) -> (error out=w360:errorcluster, "Acquisition"=w359:refnum<k24>)  [unwired: 1 out]
        n219 = property class="Bool"(reference=w346, "Disabled"=u8 0 ("Deaktiviert")) -> ()  [unwired: 1 in, 2 out]
        n220 = property class="Bool"(reference=w345, "Disabled"=u8 2 ("Deaktiviert")) -> ()  [unwired: 1 in, 2 out]
        n221 = invoke class="Acquisition" method="HasStarted"(reference=w359, error in=w360) -> (reference out=w353:refnum<k24>, error out=w356:errorcluster, "bValue"=w358:bool)  [unwired: 2 in, 1 out]
        n222 = invoke class="Acquisition" method="ToString"(reference=w353, error in=w356) -> (error out=w355:errorcluster, "ToString"=w354:string)  [unwired: 1 in, 1 out]
        n223 = call <instrlib>:"Error_Handling.vi"("Error String"=w354, "Error In"=w355) -> ("Error Out"=w357:errorcluster)  [unwired: 9 in]
        n224 = case shown="True" w358 {
          tunnel: [w370 w379] -> w349
          tunnel: w357 -> [w370 w380]
          tunnel: w351 -> [w369 w371]
          tunnel: [w369 w371] -> w350
          frame False {
          }
          frame True {
            n225 = property class="Camera"(reference=w371, error in=w380) -> (error out=w375:errorcluster, "Acquisition"=w376:refnum<k24>)  [unwired: 1 out]
            n226 = invoke class="Acquisition" method="Stop"(reference=w376, error in=w375) -> (reference out=w373:refnum<k24>, error out=w374:errorcluster, "Stop"=w372:i32)  [unwired: 1 in]
            n227 = invoke class="Acquisition" method="ToString"(reference=w373, error in=w374) -> (error out=w378:errorcluster, "ToString"=w377:string)  [unwired: 1 in, 1 out]
            n228 = call <instrlib>:"Error_Handling.vi"("Error Code"=w372, "Error String"=w377, "Error In"=w378) -> ("Error Out"=w379:errorcluster)  [unwired: 8 in]
          }
        }
        n229 = invoke class="Camera" method="Exit"(reference=w350, error in=w349) -> (reference out=w361:refnum<k24>, error out=w365:errorcluster, "Exit"=w364:i32)  [unwired: 1 in]
        n230 = invoke class="Camera" method="ToString"(reference=w361, error in=w365) -> (error out=w366:errorcluster, "ToString"=w367:string)  [unwired: 1 in, 1 out]
        n231 = call <instrlib>:"Error_Handling.vi"("Error Code"=w364, "Error String"=w367, "Error In"=w366) -> ("Error Out"=w363:errorcluster)  [unwired: 8 in]
        n232 = Close Reference ("Close Referenz")(reference=w361, error in (no error)=w363) -> (error out=w362:errorcluster)
      }
      frame Default {
        # "Has acquisition started?"
        # "Show Image"
        n233 = property class="Camera"(reference=w382, error in=w381) -> (error out=w393:errorcluster, "Acquisition"=w392:refnum<k24>)  [unwired: 1 out]
        n234 = invoke class="Acquisition" method="HasStarted"(reference=w392, error in=w393) -> (reference out=w388:refnum<k24>, error out=w387:errorcluster, "HasStarted"=w386:i32, "bValue"=w391:bool)  [unwired: 2 in]
        n235 = invoke class="Acquisition" method="ToString"(reference=w388, error in=w387) -> (error out=w390:errorcluster, "ToString"=w389:string)  [unwired: 1 in, 1 out]
        n236 = call <instrlib>:"Error_Handling.vi"("Error Code"=w386, "Error String"=w389, "Error In"=w390) -> ("Error Out"=w385:errorcluster)  [unwired: 8 in]
        n237 = case shown="False" w391 {
          tunnel: [w396 w402] -> w383
          tunnel: w385 -> [w396 w401]
          tunnel: w382 -> [w395 w397]
          tunnel: [w395 w397] -> w384
          frame False {
          }
          frame True {
            # "Memory"
            n238 = property class="Camera"(reference=w397, error in=w401) -> (error out=w404:errorcluster, "Memory"=w405:refnum<k24>)  [unwired: 1 out]
            n239 = invoke class="Memory" method="GetActive"(reference=w405, error in=w404) -> (reference out=w411:refnum<k24>, error out=w410:errorcluster, "GetActive"=w412:i32, "s32MemId"=w403:i32)  [unwired: 2 in]
            n240 = invoke class="Memory" method="ToString"(reference=w411, error in=w410) -> (error out=w408:errorcluster, "ToString"=w409:string)  [unwired: 1 in, 1 out]
            n241 = call <instrlib>:"Error_Handling.vi"("Error Code"=w412, "Error String"=w409, "Error In"=w408) -> ("Error Out"=w413:errorcluster)  [unwired: 8 in]
            n242 = property class="Camera"(reference=w397, error in=w413) -> (error out=w407:errorcluster, "Memory"=w406:refnum<k24>)  [unwired: 1 out]
            n243 = invoke class="Memory" method="CopyToArray"(reference=w406, error in=w407, "s32MemId"=w403) -> (reference out=w416:refnum<k24>, error out=w417:errorcluster, "CopyToArray"=w418:i32, "u8Image"=w398:u8[])  [unwired: 2 in, 1 out]
            n244 = invoke class="Memory" method="ToString"(reference=w416, error in=w417) -> (error out=w414:errorcluster, "ToString"=w415:string)  [unwired: 1 in, 1 out]
            n245 = call <instrlib>:"Error_Handling.vi"("Error Code"=w418, "Error String"=w415, "Error In"=w414) -> ("Error Out"=w399:errorcluster)  [unwired: 8 in]
            n246 = call <instrlib>:"ArrayToImage.vi"("Error In"=w399, "InArray"=w398, ".NET (Reference)"=w397) -> ("Error Out"=w402:errorcluster, "Image"=→"Image second camera":picture)  [unwired: 7 in]
          }
        }
      }
      frame "Init camera" {
        w427 = 1 items=["IS_DONT_WAIT", "IS_WAIT"] ("Wait")
        w454 = 0 items=["RGB 32"=0, "RGB 24"=1, "Y8 Monochrom"=6] ("Mode")
        # "SubVI Example for \nGetDefault Timing"
        # "SubVI Example for \nMemory allocation"
        # "SubVI Example for \nTiming"
        # "SubVI Example for \nCamera Init"
        # "Pixelformat"
        n247 = control-ref of="Init Camera 2"() -> (w422:refnum<vi>)
        n248 = control-ref of="Exit Camera 2"() -> (w420:refnum<vi>)
        n249 = property class="Bool"(reference=w422, "Disabled"=u8 2 ("Deaktiviert")) -> ()  [unwired: 1 in, 2 out]
        n250 = property class="Bool"(reference=w420, "Disabled"=u8 0 ("Deaktiviert")) -> ()  [unwired: 1 in, 2 out]
        n251 = call <instrlib>:"SubVI_Example_CameraInit.vi"("Error In"=w446, "Camera ID"="Camera ID 3", "Init Camera Flag"=TRUE, ".NET (Reference)"=w447) -> ("Error Out"=w451:errorcluster, ".NET (Reference)"=w425:refnum<k24>)  [unwired: 6 in]
        n252 = property class="Camera"(reference=w425, error in=w451) -> (error out=w452:errorcluster, "PixelFormat"=w453:refnum<k24>)  [unwired: 1 out]
        n253 = invoke class="PixelFormat" method="Set"(reference=w453, error in=w452, "mode"=w454) -> (reference out=w449:refnum<k24>, error out=w443:errorcluster, "Set"=w448:i32)  [unwired: 1 in, 1 out]
        n254 = invoke class="PixelFormat" method="ToString"(reference=w449, error in=w443) -> (error out=w442:errorcluster, "ToString"=w450:string)  [unwired: 1 in, 1 out]
        n255 = call <instrlib>:"Error_Handling.vi"("Error Code"=w448, "Error String"=w450, "Error In"=w442) -> ("Error Out"=w439:errorcluster)  [unwired: 8 in]
        n256 = call <instrlib>:"SubVI_Example_GetDefault_Timing.vi"(".NET (Reference)"=w425, "Error In"=w439) -> ("Pixelclock"=w436:i32, "Exposure time"=w437:dbl, "Framerate"=w438:dbl, "Error Out"=w435:errorcluster)  [unwired: 10 in]
        n257 = call <instrlib>:"SubVI_Example_Timing.vi"(".NET (Reference)"=w425, "Pixelclock"=w436, "Exposure time"=w437, "Framerate"=w438, "Error In"=w435) -> ("Error Out"=w441:errorcluster)  [unwired: 7 in, 3 out]
        n258 = call <instrlib>:"SubVI_Example_MemoryAllocation.vi"(".NET (Reference)"=w425, "Error In"=w441) -> ("Serial Number"=→"Serial Number 2":string, "Error Out"=w424:errorcluster)  [unwired: 13 in, 3 out]
        n259 = property class="Camera"(reference=w425, error in=w424) -> (error out=w433:errorcluster, "Acquisition"=w434:refnum<k24>)  [unwired: 1 out]
        n260 = invoke class="Acquisition" method="Capture"(reference=w434, error in=w433, "param"=w427) -> (reference out=w429:refnum<k24>, error out=w430:errorcluster, "Capture"=w428:i32)  [unwired: 1 in, 1 out]
        n261 = invoke class="Acquisition" method="ToString"(reference=w429, error in=w430) -> (error out=w432:errorcluster, "ToString"=w431:string)  [unwired: 1 in, 1 out]
        n262 = call <instrlib>:"Error_Handling.vi"("Error Code"=w428, "Error String"=w431, "Error In"=w432) -> ("Error Out"=w426:errorcluster)  [unwired: 8 in]
      }
    }
    n263 = case shown="Default" w222 {
      tunnel: w213 -> [w465 w496 w561]
      tunnel: w212 -> [w466 w495 w560]
      tunnel: [w475 w498 w540] -> w215
      tunnel: [w476 w497 w541] -> w219
      tunnel: [TRUE FALSE FALSE] -> w217
      frame "Exit camera" {
        # "Close .Net Referenz"
        # "Is acquisition running?"
        # "Stop Acquisition"
        # "Close Camera"
        n264 = control-ref of="Init Camera"() -> (w460:refnum<vi>)
        n265 = control-ref of="Exit Camera"() -> (w459:refnum<vi>)
        n266 = property class="Camera"(reference=w465, error in=w466) -> (error out=w474:errorcluster, "Acquisition"=w473:refnum<k24>)  [unwired: 1 out]
        n267 = property class="Bool"(reference=w460, "Disabled"=u8 0 ("Deaktiviert")) -> ()  [unwired: 1 in, 2 out]
        n268 = property class="Bool"(reference=w459, "Disabled"=u8 2 ("Deaktiviert")) -> ()  [unwired: 1 in, 2 out]
        n269 = invoke class="Acquisition" method="HasStarted"(reference=w473, error in=w474) -> (reference out=w467:refnum<k24>, error out=w470:errorcluster, "bValue"=w472:bool)  [unwired: 2 in, 1 out]
        n270 = invoke class="Acquisition" method="ToString"(reference=w467, error in=w470) -> (error out=w469:errorcluster, "ToString"=w468:string)  [unwired: 1 in, 1 out]
        n271 = call <instrlib>:"Error_Handling.vi"("Error String"=w468, "Error In"=w469) -> ("Error Out"=w471:errorcluster)  [unwired: 9 in]
        n272 = case shown="True" w472 {
          tunnel: [w484 w493] -> w463
          tunnel: w471 -> [w484 w494]
          tunnel: w465 -> [w483 w485]
          tunnel: [w483 w485] -> w464
          frame False {
          }
          frame True {
            n273 = property class="Camera"(reference=w485, error in=w494) -> (error out=w489:errorcluster, "Acquisition"=w490:refnum<k24>)  [unwired: 1 out]
            n274 = invoke class="Acquisition" method="Stop"(reference=w490, error in=w489) -> (reference out=w487:refnum<k24>, error out=w488:errorcluster, "Stop"=w486:i32)  [unwired: 1 in]
            n275 = invoke class="Acquisition" method="ToString"(reference=w487, error in=w488) -> (error out=w492:errorcluster, "ToString"=w491:string)  [unwired: 1 in, 1 out]
            n276 = call <instrlib>:"Error_Handling.vi"("Error Code"=w486, "Error String"=w491, "Error In"=w492) -> ("Error Out"=w493:errorcluster)  [unwired: 8 in]
          }
        }
        n277 = invoke class="Camera" method="Exit"(reference=w464, error in=w463) -> (reference out=w475:refnum<k24>, error out=w479:errorcluster, "Exit"=w478:i32)  [unwired: 1 in]
        n278 = invoke class="Camera" method="ToString"(reference=w475, error in=w479) -> (error out=w480:errorcluster, "ToString"=w481:string)  [unwired: 1 in, 1 out]
        n279 = call <instrlib>:"Error_Handling.vi"("Error Code"=w478, "Error String"=w481, "Error In"=w480) -> ("Error Out"=w477:errorcluster)  [unwired: 8 in]
        n280 = Close Reference ("Close Referenz")(reference=w475, error in (no error)=w477) -> (error out=w476:errorcluster)
      }
      frame Default {
        # "Has acquisition started?"
        n281 = property class="Camera"(reference=w496, error in=w495) -> (error out=w507:errorcluster, "Acquisition"=w506:refnum<k24>)  [unwired: 1 out]
        n282 = invoke class="Acquisition" method="HasStarted"(reference=w506, error in=w507) -> (reference out=w502:refnum<k24>, error out=w501:errorcluster, "HasStarted"=w500:i32, "bValue"=w505:bool)  [unwired: 2 in]
        n283 = invoke class="Acquisition" method="ToString"(reference=w502, error in=w501) -> (error out=w504:errorcluster, "ToString"=w503:string)  [unwired: 1 in, 1 out]
        n284 = call <instrlib>:"Error_Handling.vi"("Error Code"=w500, "Error String"=w503, "Error In"=w504) -> ("Error Out"=w499:errorcluster)  [unwired: 8 in]
        n285 = case shown="True" w505 {
          tunnel: [w510 w516] -> w497
          tunnel: w499 -> [w510 w515]
          tunnel: w496 -> [w509 w513]
          tunnel: [w509 w513] -> w498
          frame False {
            # "Show Image"
          }
          frame True {
            # "Memory"
            n286 = property class="Camera"(reference=w513, error in=w515) -> (error out=w518:errorcluster, "Memory"=w519:refnum<k24>)  [unwired: 1 out]
            n287 = invoke class="Memory" method="GetActive"(reference=w519, error in=w518) -> (reference out=w525:refnum<k24>, error out=w524:errorcluster, "GetActive"=w526:i32, "s32MemId"=w517:i32)  [unwired: 2 in]
            n288 = invoke class="Memory" method="ToString"(reference=w525, error in=w524) -> (error out=w522:errorcluster, "ToString"=w523:string)  [unwired: 1 in, 1 out]
            n289 = call <instrlib>:"Error_Handling.vi"("Error Code"=w526, "Error String"=w523, "Error In"=w522) -> ("Error Out"=w527:errorcluster)  [unwired: 8 in]
            n290 = property class="Camera"(reference=w513, error in=w527) -> (error out=w521:errorcluster, "Memory"=w520:refnum<k24>)  [unwired: 1 out]
            n291 = invoke class="Memory" method="CopyToArray"(reference=w520, error in=w521, "s32MemId"=w517) -> (reference out=w530:refnum<k24>, error out=w531:errorcluster, "CopyToArray"=w532:i32, "u8Image"=w512:u8[])  [unwired: 2 in, 1 out]
            n292 = invoke class="Memory" method="ToString"(reference=w530, error in=w531) -> (error out=w528:errorcluster, "ToString"=w529:string)  [unwired: 1 in, 1 out]
            n293 = call <instrlib>:"Error_Handling.vi"("Error Code"=w532, "Error String"=w529, "Error In"=w528) -> ("Error Out"=w514:errorcluster)  [unwired: 8 in]
            n294 = call <instrlib>:"ArrayToImage.vi"("Error In"=w514, "InArray"=w512, ".NET (Reference)"=w513) -> ("Error Out"=w516:errorcluster, "Image"=→"Image first camera":picture)  [unwired: 7 in]
          }
        }
      }
      frame "Init camera" {
        w542 = 1 items=["IS_DONT_WAIT", "IS_WAIT"] ("Wait")
        w568 = 0 items=["RGB 32"=0, "RGB 24"=1, "Y8 Monochrom"=6] ("Mode")
        # "SubVI Example for \nGetDefault Timing"
        # "SubVI Example for \nMemory allocation"
        # "SubVI Example for \nTiming"
        # "SubVI Example for \nCamera Init"
        # "Pixelformat"
        n295 = control-ref of="Init Camera"() -> (w536:refnum<vi>)
        n296 = control-ref of="Exit Camera"() -> (w534:refnum<vi>)
        n297 = call <instrlib>:"SubVI_Example_CameraInit.vi"("Error In"=w560, "Camera ID"="Camera ID 1", "Init Camera Flag"=TRUE, ".NET (Reference)"=w561) -> ("Error Out"=w565:errorcluster, ".NET (Reference)"=w540:refnum<k24>)  [unwired: 6 in]
        n298 = property class="Bool"(reference=w536, "Disabled"=u8 2 ("Deaktiviert")) -> ()  [unwired: 1 in, 2 out]
        n299 = property class="Bool"(reference=w534, "Disabled"=u8 0 ("Deaktiviert")) -> ()  [unwired: 1 in, 2 out]
        n300 = property class="Camera"(reference=w540, error in=w565) -> (error out=w566:errorcluster, "PixelFormat"=w567:refnum<k24>)  [unwired: 1 out]
        n301 = invoke class="PixelFormat" method="Set"(reference=w567, error in=w566, "mode"=w568) -> (reference out=w563:refnum<k24>, error out=w557:errorcluster, "Set"=w562:i32)  [unwired: 1 in, 1 out]
        n302 = invoke class="PixelFormat" method="ToString"(reference=w563, error in=w557) -> (error out=w556:errorcluster, "ToString"=w564:string)  [unwired: 1 in, 1 out]
        n303 = call <instrlib>:"Error_Handling.vi"("Error Code"=w562, "Error String"=w564, "Error In"=w556) -> ("Error Out"=w553:errorcluster)  [unwired: 8 in]
        n304 = call <instrlib>:"SubVI_Example_GetDefault_Timing.vi"(".NET (Reference)"=w540, "Error In"=w553) -> ("Pixelclock"=w550:i32, "Exposure time"=w551:dbl, "Framerate"=w552:dbl, "Error Out"=w538:errorcluster)  [unwired: 10 in]
        n305 = call <instrlib>:"SubVI_Example_Timing.vi"(".NET (Reference)"=w540, "Pixelclock"=w550, "Exposure time"=w551, "Framerate"=w552, "Error In"=w538) -> ("Error Out"=w555:errorcluster)  [unwired: 7 in, 3 out]
        n306 = call <instrlib>:"SubVI_Example_MemoryAllocation.vi"(".NET (Reference)"=w540, "Error In"=w555) -> ("Serial Number"=→"Serial Number 1":string, "Error Out"=w539:errorcluster)  [unwired: 13 in, 3 out]
        n307 = property class="Camera"(reference=w540, error in=w539) -> (error out=w548:errorcluster, "Acquisition"=w549:refnum<k24>)  [unwired: 1 out]
        n308 = invoke class="Acquisition" method="Capture"(reference=w549, error in=w548, "param"=w542) -> (reference out=w544:refnum<k24>, error out=w545:errorcluster, "Capture"=w543:i32)  [unwired: 1 in, 1 out]
        n309 = invoke class="Acquisition" method="ToString"(reference=w544, error in=w545) -> (error out=w547:errorcluster, "ToString"=w546:string)  [unwired: 1 in, 1 out]
        n310 = call <instrlib>:"Error_Handling.vi"("Error Code"=w543, "Error String"=w546, "Error In"=w547) -> ("Error Out"=w541:errorcluster)  [unwired: 8 in]
      }
    }
    n311 = case shown="False" "steps /\n continuous \ntoggle" {
      tunnel: w186 -> [w243 w319]
      tunnel: w185 -> [w242 w318]
      tunnel: [w261 w325] -> w184
      tunnel: [w234 w331] -> w174
      tunnel: "up a1" -> [w260 w327]
      tunnel: "down a1" -> [w258 w326]
      tunnel: "up all" -> [w241 w314]
      tunnel: "down all" -> [w240 w315]
      tunnel: "down a3" -> [w248 w323]
      tunnel: "up a3" -> [w249 w322]
      tunnel: "down a2" -> [w246 w317]
      tunnel: "up a2" -> [w247 w316]
      tunnel: w179 -> [_ w329]
      tunnel: [_ w330] -> w183
      tunnel: [_ w310] -> w182
      tunnel: w178 -> [_ w307]
      tunnel: [_ w308] -> w180
      tunnel: w176 -> [_ w305]
      tunnel: [_ w309] -> w181
      tunnel: w177 -> [_ w306]
      frame False {
        n312 = flat-sequence {
          tunnel: w243 -> [w276]
          tunnel: w242 -> [w279]
          tunnel: w249 -> [w274]
          tunnel: "a3" ("Combo Box") -> [w272]
          tunnel: "Step size" -> [w275]
          tunnel: w248 -> [w273]
          tunnel: [w278] -> w252
          tunnel: [w277] -> w251
          tunnel: [w281] -> _
          tunnel: [w282] -> w236
          tunnel: w252 -> [w282]
          tunnel: w251 -> [w281]
          frame #0 {
            n313 = call "Picomotor step single.vi"("Step size"=w275, "Combo Box"=w272, "error in (no error)"=w279, "down a1"=w273, "up a1"=w274, "VISA Refnum in"=w276) -> ("error out"=w278:errorcluster, "VISA Refnum out"=w277:refnum<visa-resource-name>)  [unwired: 4 in]
          }
          frame #1 {
            n314 = Wait (ms)(milliseconds to wait=u32 100) -> ()  [unwired: 1 out]
          }
        }
        n315 = flat-sequence {
          tunnel: w243 -> [w298]
          tunnel: w242 -> [w301]
          tunnel: w260 -> [w296]
          tunnel: "a1" ("Combo Box") -> [w294]
          tunnel: "Step size" -> [w297]
          tunnel: w258 -> [w295]
          tunnel: [w300] -> w257
          tunnel: [w299] -> w256
          tunnel: [w303] -> w261
          tunnel: [w304] -> w238
          tunnel: w257 -> [w304]
          tunnel: w256 -> [w303]
          frame #0 {
            n316 = call "Picomotor step single.vi"("Step size"=w297, "Combo Box"=w294, "error in (no error)"=w301, "down a1"=w295, "up a1"=w296, "VISA Refnum in"=w298) -> ("error out"=w300:errorcluster, "VISA Refnum out"=w299:refnum<visa-resource-name>)  [unwired: 4 in]
          }
          frame #1 {
            n317 = Wait (ms)(milliseconds to wait=u32 100) -> ()  [unwired: 1 out]
          }
        }
        n318 = flat-sequence {
          tunnel: w243 -> [w287]
          tunnel: w242 -> [w290]
          tunnel: w247 -> [w285]
          tunnel: "a2" ("Combo Box") -> [w283]
          tunnel: "Step size" -> [w286]
          tunnel: w246 -> [w284]
          tunnel: [w289] -> w255
          tunnel: [w288] -> w254
          tunnel: [w292] -> _
          tunnel: [w293] -> w237
          tunnel: w255 -> [w293]
          tunnel: w254 -> [w292]
          frame #0 {
            n319 = call "Picomotor step single.vi"("Step size"=w286, "Combo Box"=w283, "error in (no error)"=w290, "down a1"=w284, "up a1"=w285, "VISA Refnum in"=w287) -> ("error out"=w289:errorcluster, "VISA Refnum out"=w288:refnum<visa-resource-name>)  [unwired: 4 in]
          }
          frame #1 {
            n320 = Wait (ms)(milliseconds to wait=u32 100) -> ()  [unwired: 1 out]
          }
        }
        n321 = flat-sequence {
          tunnel: [w268] -> w245
          tunnel: [w267] -> w244
          tunnel: w243 -> [w266]
          tunnel: w242 -> [w265]
          tunnel: w241 -> [w264]
          tunnel: w240 -> [w263]
          tunnel: "Step size" -> [w262]
          tunnel: [w270] -> _
          tunnel: [w271] -> w235
          tunnel: w245 -> [w271]
          tunnel: w244 -> [w270]
          frame #0 {
            n322 = call "Picomotor step multi.vi"("Step size"=w262, "error in (no error)"=w265, "down a1"=w263, "up a1"=w264, "VISA Refnum in"=w266) -> ("error out"=w268:errorcluster, "VISA Refnum out"=w267:refnum<visa-resource-name>)  [unwired: 5 in]
          }
          frame #1 {
            n323 = Wait (ms)(milliseconds to wait=u32 100) -> ()  [unwired: 1 out]
          }
        }
        n324 = Merge Errors(w238, w237, w236, w235) -> (w234:errorcluster)
      }
      frame True {
        n325 = call "Picomotor single motor continuous.vi"("Enum"=w329, "Combo Box"="a1", "error in (no error)"=w318, "down"=w326, "up"=w327, "VISA Refnum in"=w319) -> ("error out"=w324:errorcluster, "Numeric"=w330:i32, "VISA Refnum out"=w325:refnum<visa-resource-name>)  [unwired: 3 in]
        n326 = call "Picomotor single motor continuous.vi"("Enum"=w306, "Combo Box"="a3", "error in (no error)"=w318, "down"=w323, "up"=w322, "VISA Refnum in"=w319) -> ("error out"=w312:errorcluster, "Numeric"=w309:i32)  [unwired: 3 in, 1 out]
        n327 = call "Picomotor single motor continuous.vi"("Enum"=w307, "Combo Box"="a2", "error in (no error)"=w318, "down"=w317, "up"=w316, "VISA Refnum in"=w319) -> ("error out"=w313:errorcluster, "Numeric"=w310:i32)  [unwired: 3 in, 1 out]
        n328 = call "Picomotor all motors continuous.vi"("Enum"=w305, "error in (no error)"=w318, "down"=w315, "up"=w314, "VISA Refnum in"=w319) -> ("error out"=w311:errorcluster, "Numeric"=w308:i32)  [unwired: 4 in, 1 out]
        n329 = Merge Errors(w324, w313, w312, w311) -> (w331:errorcluster)
      }
    }
    n330 = call <instrlib>:"SubVI_Example_SyncEventLoop.vi"("Error In"=w206, "use sync"=w204, ".NET (Reference)"=w202) -> ("Error Out"=w201:errorcluster, "Synchronize (ms)"=w205:dbl)  [unwired: 7 in]
    "Error Camera 2" <- w201
    n331 = call <instrlib>:"SubVI_Example_SyncEventLoop.vi"("Error In"=w219, "use sync"=w217, ".NET (Reference)"=w215) -> ("Error Out"=w214:errorcluster, "Synchronize (ms)"=w218:dbl)  [unwired: 7 in]
    "Error Camera 1" <- w214
    n332 = Wait Until Next ms Multiple(millisecond multiple=w218) -> ()  [unwired: 1 out]
    n333 = Wait Until Next ms Multiple(millisecond multiple=w205) -> ()  [unwired: 1 out]
    n334 = case shown="True" "stop" {
      tunnel: w184 -> [w334 w339]
      tunnel: w174 -> [w333 w338]
      tunnel: [w334 w337] -> w173
      tunnel: [w333 w336] -> w175
      tunnel: [w332 w335] -> w197
      tunnel: "stop" -> [w332 w335]
      frame False {
      }
      frame True {
        n335 = call "Picomotor Write.vi"("error in (no error)"=w338, "String 3"="sto", "VISA Refnum in"=w339) -> ("error out"=w336:errorcluster, "VISA Refnum out"=w337:refnum<visa-resource-name>)  [unwired: 6 in, 1 out]
      }
    }
    n336 = Merge Errors(w175, w174) -> (w198:errorcluster)
  }
  n337 = VISA Close(VISA resource name=w1, error in (no error)=w2) -> (error out=→"error":errorcluster)
